vi "Periodic Tasks.vi"(8 "error in":errorcluster) -> ()   [LabVIEW 2020]
doc: "This VI runs in parallel to other tasks. It can contain as many user-defined periodic loops as you need. These can carry out PID or other sorts of timed response."
uses:
  <vilib>/Rock Robotics/WPI/ThirdParty/Phoenix-LabVIEW/Motor Controller/Controls/CTRE_Phoenix_MotorControl_ControlMode.ctl
  <vilib>/Rock Robotics/WPI/Solenoid/WPI_SolenoidValue.ctl
  <vilib>/Rock Robotics/WPI/DriverStation/WPI_DriverStationAllianceInfo.ctl
  <vilib>/Rock Robotics/WPI/Utilities/WPI_GetSetVariantRefNum.vi
  Robot Global Data.vi
  <vilib>/Rock Robotics/WPI/Solenoid/WPI_SolenoidSetEnum.vi
  <vilib>/Rock Robotics/WPI/ThirdParty/Phoenix-LabVIEW/Motor Controller/Get/CTRE_Phoenix_MotorController_IntegratedSensorData_TalonFX.vi
  <vilib>/Rock Robotics/WPI/ThirdParty/Phoenix-LabVIEW/Motor Controller/Get/CTRE_Phoenix_MotorController_GetQuadratureData.vi
  <vilib>/Rock Robotics/WPI/ThirdParty/Phoenix-LabVIEW/Motor Controller/Sensor/CTRE_Phoenix_MotorControl_SetIntegratedSensorPosition_TalonFX.vi
  <vilib>/Rock Robotics/Network Tables/NT Read Numeric Array.vi
  <vilib>/Rock Robotics/Network Tables/NT Read String Array.vi
  <vilib>/Rock Robotics/Network Tables/NT Read Boolean Array.vi
  <vilib>/Rock Robotics/Network Tables/NT Write String Array.vi
  <vilib>/Rock Robotics/Network Tables/NT Write Boolean Array.vi
  <vilib>/Rock Robotics/Network Tables/NT Write Numeric Array.vi
  <vilib>/Rock Robotics/Network Tables/NT Read Number.vi
  <vilib>/Rock Robotics/Network Tables/NT Write Number.vi
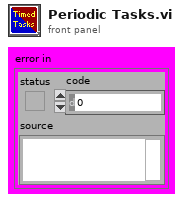
[diagram p1: front panel]
types:
  T1 = enum16{"Do Nothing", "Cargo", "Low", "High", "Long Shot", "U", "Hook", "Tee", "Eject"}
  T2 = enum16{"Do Nothing", "Cargo", "Low", "High", "Long Shot", "U", "Hook", "Tee"}
  T3 = typedef "WPI_GyroDevRef.ctl" = cluster{"DevStatus":errorcluster, "Analog Channel":T4, "Gain (VoltsPerDegree/Second)":dbl, "Gyro Type":enum16{"Analog", "XRS450"}, "Handle":i32, "SPI Bus":T5, "Device Found":bool, "Sample Rate":dbl, "Calibrate On Open":bool, "Offset":dbl}
  T4 = typedef "FPGA_AIChannel.ctl" = enum8{"AI 0", "AI 1", "AI 2", "AI 3", "AI MXP 0", "AI MXP 1", "AI MXP 2", "AI MXP 3", "Invalid"}
  T5 = typedef "spi_bus.ctl" = enum16{"SPI On-Board, CS0", "SPI On-Board, CS1", "SPI On-Board, CS2", "SPI On-Board, CS3", "SPI MXP", "Invalid"}
  T6 = typedef "WPI_PotentiometerDevRef.ctl" = cluster{"DevStatus":errorcluster, "Analog Channel":T4, "Invert Output":bool}
  T7 = typedef "WPI_DigitalInputDevRef.ctl" = cluster{"DevStatus":errorcluster, "DIO Channel":T8}
  T8 = typedef "FPGA_DIOChannel.ctl" = enum8{"DIO 0", "DIO 1", "DIO 2", "DIO 3", "DIO 4", "DIO 5", "DIO 6", "DIO 7", "DIO 8", "DIO 9", "DIO MXP 0", "DIO MXP 1", "DIO MXP 2", "DIO MXP 3", "DIO MXP 4", "DIO MXP 5", "DIO MXP 6", "DIO MXP 7", "DIO MXP 8", "DIO MXP 9", "DIO MXP 10", "DIO MXP 11", "DIO MXP 12", "DIO MXP 13", "DIO MXP 14", "DIO MXP 15", "SPI Port CS1", "SPI Port CS2", "SPI Port CS3", "SPI Port MISO", "SPI Port MOSI", "Invalid"}
  T9 = typedef "WPI_SolenoidDevRef.ctl" = cluster{"DevStatus":errorcluster, "Pneumatics Control Module":u8, "Forward Solenoid Channel":T10, "Reverse Solenoid Channel":T10}
  T10 = typedef "WPI_SolenoidChannel.ctl" = enum8{"Solenoid 0", "Solenoid 1", "Solenoid 2", "Solenoid 3", "Solenoid 4", "Solenoid 5", "Solenoid 6", "Solenoid 7", "Solenoid 8", "Solenoid 9", "Solenoid 10", "Solenoid 11", "Solenoid 12", "Solenoid 13", "Solenoid 14", "Solenoid 15", "Invalid"}
  T11 = typedef "WPI_SolenoidValue.ctl" = enum16{"Off", "On", "Forward", "Reverse"}
  T12 = typedef "WPI_AnalogChannelDevRef.ctl" = cluster{"DevStatus":errorcluster, "Analog Channel":T4}
  T13 = typedef "WPI_JoystickDevRef.ctl" = cluster{"Device":T14}
  T14 = typedef "WPI_JoystickDeviceEnum.ctl" = enum16{"USB 0", "USB 1", "USB 2", "USB 3", "USB 4", "USB 5"}
  T15 = typedef "WPI_MotorControlDeviceRef.ctl" = cluster{"DeviceStatus":errorcluster, "Type":T16, "PWM":cluster{"PWM Channel":T17, "DeadBand":T18}, "CAN":cluster{"Device Number":u8, "SetOutput VI Ref":variant, "GetOutput VI Ref":variant, "Enable VI Ref":variant, "Disable VI Ref":variant, "Data":variant}, "Invert":bool, "DIO PWM":cluster{"PWM \"Enable\" Channel":T17, "DIOChannel":T8, "PWM Rate":dbl}}
  T16 = typedef "WPI_MotorControlType.ctl" = enum16{"PWM", "CAN", "DIO PWM"}
  T17 = typedef "FPGA_DIOPWMChannel.ctl" = enum8{"PWM 0", "PWM 1", "PWM 2", "PWM 3", "PWM 4", "PWM 5", "PWM 6", "PWM 7", "PWM 8", "PWM 9", "PWM MXP 0", "PWM MXP 1", "PWM MXP 2", "PWM MXP 3", "PWM MXP 4", "PWM MXP 5", "PWM MXP 6", "PWM MXP 7", "PWM MXP 8", "PWM MXP 9", "Invalid"}
  T18 = typedef "WPI_PWMDeadband.ctl" = cluster{"Name":string, "maxPositivePwm":i32, "minPositivePwm":i32, "centerPwm":i32, "maxNegativePwm":i32, "minNegativePwm":i32, "angularRange":u16}
  T19 = typedef "CTRE_Phoenix_MotorControl_ControlMode.ctl" = u16
  T20 = typedef "WPI_RobotDriveDevRef.ctl" = cluster{"DevStatus":errorcluster, "Motors[]":T15[], "Square Inputs":bool, "Max Output":dbl}
  T21 = cluster{"JoystickDevRef":T13, "RobotDriveDevRef":T20}
  T22 = typedef "WPI_DigitalOutputDevRef.ctl" = cluster{"DIO Channel":T8, "DevStatus":errorcluster}
  T23 = typedef "WPI_DriverStationAllianceInfo.ctl" = enum16{"Red", "Blue", "Invalid"}
  T24 = typedef "WPI_RelayDevRef.ctl" = cluster{"DevStatus":errorcluster, "Relay Channel":T25, "Relay Direction":T26}
  T25 = typedef "FPGA_DIORelayChannel.ctl" = enum8{"Relay 0", "Relay 1", "Relay 2", "Relay 3", "Invalid"}
  T26 = typedef "WPI_RelayDirection.ctl" = enum16{"Both directions", "Forward only", "Reverse only"}
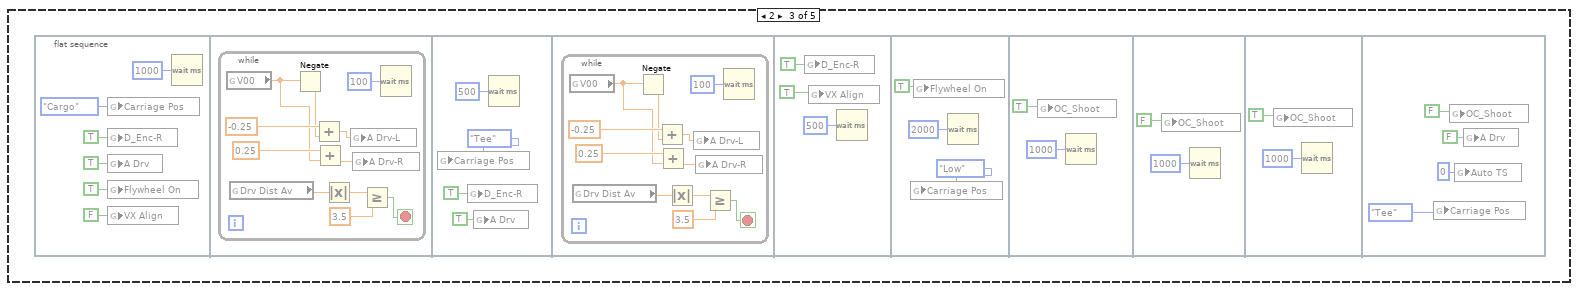
[diagram p13: hidden frame]
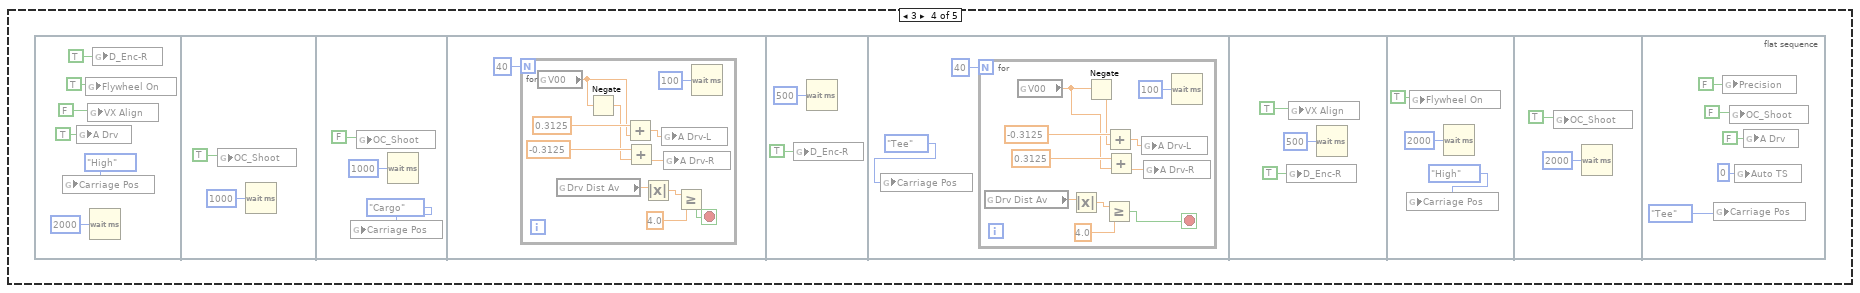
[diagram p14: hidden frame]
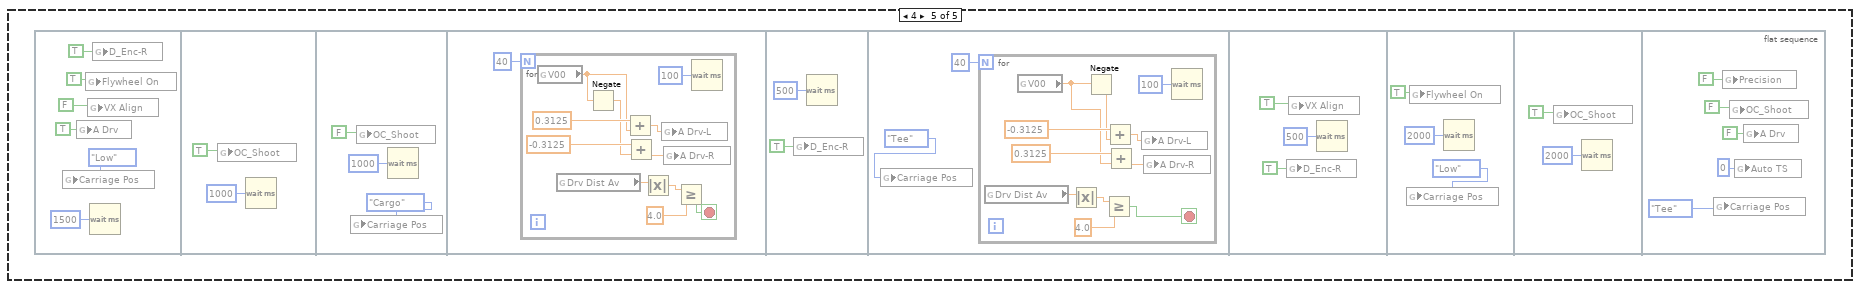
[diagram p15: hidden frame]
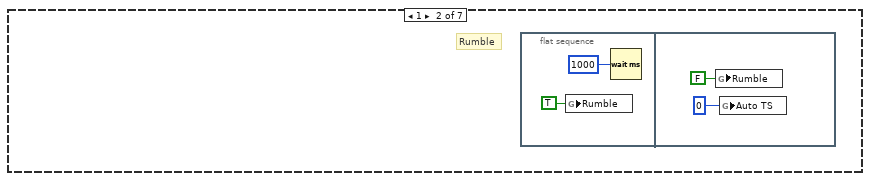
[diagram p18: hidden frame]
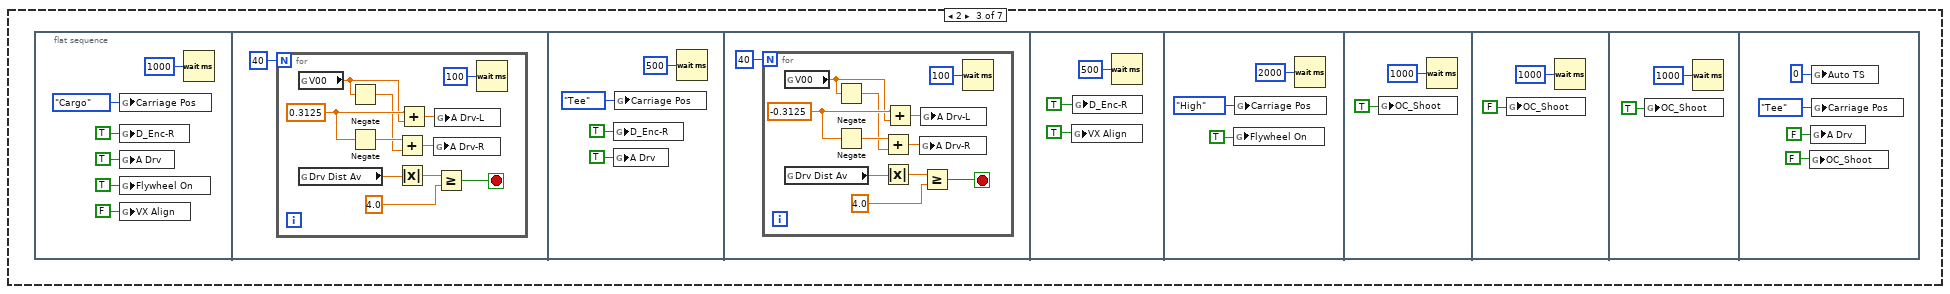
[diagram p19: hidden frame]
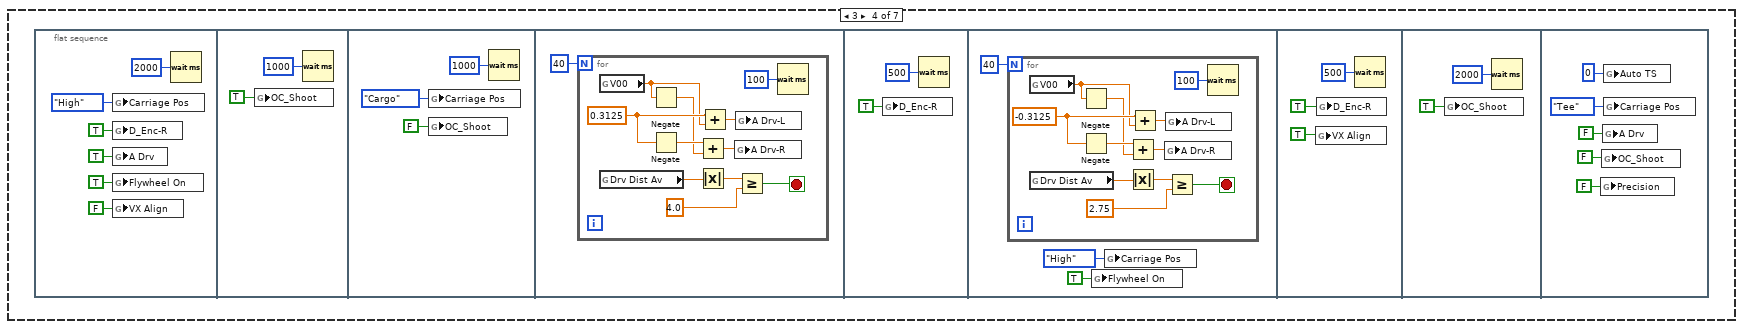
[diagram p20: hidden frame]
diagram:
  (unwired) "This VI is a good place to take care of periodic tasks such as control loops.\n\nAdd code to the existing loops, or duplicate a loop to define a new rate. You can allocate I/O references here, or in Begin.vi.\n\nPeriodic loops will often operate with setpoints from other loops. Use a global variable such as Robot Global Data for sharing data between loops."
  # "Autonomous\nTiming Sequence\n[Precondition: Tee Position]\n2 - Prep to pickup Cargo \nMove out of Tarmac to get one Cargo \nMove back into Tarmac to initial position \nMake two High Shots\n\n[Precondition: U Position]\n3 - Move to High position;\nMake one High Shot \nPrep to pickup Cargo \nMove out of  Tarmac to get one Cargo \nMove back into Tarmac to initial position  \nMake one High Shot\n\n[Precondition: U or Low Position]\n4 - Move to Low Position \nMake one Low Shot \nPrep to pickup Cargo \nMove out of Tarmac to get one Cargo \nMove back into Tarmac to initial position\nMake one Low Shot"
  # "Old Autonomous Sequences;\nStill works just is messy"
  # "s"
  n1 = disable-structure shown="Disabled" {
    frame Disabled {
      n2 = while {
        stop <- FALSE stop-if-true
        # "Autonomous\nTiming Sequence\n0 - Do Nothing\n1 - Rumble"
        n3 = global read "Robot Global Data.vi" "Auto TS"() -> (w39:i8)
        n4 = case shown="1" w39 {
          frame 0, Default {
            # "Do Nothing"
          }
          frame 1 {
            # "Rumble"
            n5 = flat-sequence {
              frame #0 {
                n6 = global write "Robot Global Data.vi" "Rumble"(TRUE ("Rumble")) -> ()
                n7 = Wait (ms)(milliseconds to wait=u32 1000) -> ()  [unwired: 1 out]
              }
              frame #1 {
                n8 = global write "Robot Global Data.vi" "Rumble"(FALSE ("Rumble")) -> ()
                n9 = global write "Robot Global Data.vi" "Auto TS"(i8 0 ("Autono R")) -> ()
              }
            }
          }
          frame 2 {
            n10 = flat-sequence {
              frame #0 {
                n11 = global write "Robot Global Data.vi" "Carriage Pos"(T1."Cargo" ("Carriage Pos")) -> ()
                n12 = global write "Robot Global Data.vi" "D_Enc-R"(TRUE ("D_Enc-R")) -> ()
                n13 = global write "Robot Global Data.vi" "A Drv"(TRUE ("A Drv")) -> ()
                n14 = global write "Robot Global Data.vi" "Flywheel On"(TRUE ("A Drv")) -> ()
                n15 = global write "Robot Global Data.vi" "VX Align"(FALSE ("VX Align")) -> ()
                n16 = Wait (ms)(milliseconds to wait=u32 1000) -> ()  [unwired: 1 out]
              }
              frame #1 {
                n17 = while {
                  stop <- w62 stop-if-true
                  n18 = global read "Robot Global Data.vi" "V00"() -> (w54:dbl)
                  n19 = global read "Robot Global Data.vi" "Drv Dist Av"() -> (w61:dbl)
                  n20 = Negate(x=w54) -> (-x=w53:dbl)
                  n21 = Add(x=-0.25 ("A Drv-L"), y=w53) -> (x+y=w58:dbl)
                  n22 = Add(x=0.25 ("A Drv-R"), y=w54) -> (x+y=w57:dbl)
                  n23 = Absolute Value(x=w61) -> (abs(x)=w52:dbl)
                  n24 = global write "Robot Global Data.vi" "A Drv-L"(w58) -> ()
                  n25 = global write "Robot Global Data.vi" "A Drv-R"(w57) -> ()
                  n26 = Greater Or Equal?(x=w52, y=3.5) -> (x >= y?=w62:bool)
                  n27 = Wait (ms)(milliseconds to wait=u32 100) -> ()  [unwired: 1 out]
                }
              }
              frame #2 {
                n28 = global write "Robot Global Data.vi" "Carriage Pos"(T2."Tee" ("Carriage Pos")) -> ()
                n29 = global write "Robot Global Data.vi" "D_Enc-R"(TRUE ("D_Enc-R")) -> ()
                n30 = global write "Robot Global Data.vi" "A Drv"(TRUE ("A Drv")) -> ()
                n31 = Wait (ms)(milliseconds to wait=u32 500) -> ()  [unwired: 1 out]
              }
              frame #3 {
                n32 = while {
                  stop <- w77 stop-if-true
                  n33 = global read "Robot Global Data.vi" "V00"() -> (w69:dbl)
                  n34 = global read "Robot Global Data.vi" "Drv Dist Av"() -> (w76:dbl)
                  n35 = Negate(x=w69) -> (-x=w68:dbl)
                  n36 = Add(x=-0.25 ("A Drv-L"), y=w68) -> (x+y=w73:dbl)
                  n37 = Add(x=0.25 ("A Drv-R"), y=w69) -> (x+y=w72:dbl)
                  n38 = Absolute Value(x=w76) -> (abs(x)=w67:dbl)
                  n39 = global write "Robot Global Data.vi" "A Drv-L"(w73) -> ()
                  n40 = global write "Robot Global Data.vi" "A Drv-R"(w72) -> ()
                  n41 = Greater Or Equal?(x=w67, y=3.5) -> (x >= y?=w77:bool)
                  n42 = Wait (ms)(milliseconds to wait=u32 100) -> ()  [unwired: 1 out]
                }
              }
              frame #4 {
                n43 = global write "Robot Global Data.vi" "D_Enc-R"(TRUE ("D_Enc-R")) -> ()
                n44 = global write "Robot Global Data.vi" "VX Align"(TRUE ("A Drv")) -> ()
                n45 = Wait (ms)(milliseconds to wait=u32 500) -> ()  [unwired: 1 out]
              }
              frame #5 {
                n46 = global write "Robot Global Data.vi" "Carriage Pos"(T2."Low" ("Carriage Pos")) -> ()
                n47 = global write "Robot Global Data.vi" "Flywheel On"(TRUE ("A Drv")) -> ()
                n48 = Wait (ms)(milliseconds to wait=u32 2000) -> ()  [unwired: 1 out]
              }
              frame #6 {
                n49 = global write "Robot Global Data.vi" "OC_Shoot"(TRUE ("A Drv")) -> ()
                n50 = Wait (ms)(milliseconds to wait=u32 1000) -> ()  [unwired: 1 out]
              }
              frame #7 {
                n51 = global write "Robot Global Data.vi" "OC_Shoot"(FALSE ("A Drv")) -> ()
                n52 = Wait (ms)(milliseconds to wait=u32 1000) -> ()  [unwired: 1 out]
              }
              frame #8 {
                n53 = global write "Robot Global Data.vi" "OC_Shoot"(TRUE ("A Drv")) -> ()
                n54 = Wait (ms)(milliseconds to wait=u32 1000) -> ()  [unwired: 1 out]
              }
              frame #9 {
                n55 = global write "Robot Global Data.vi" "Carriage Pos"(T2."Tee" ("Carriage Pos")) -> ()
                n56 = global write "Robot Global Data.vi" "OC_Shoot"(FALSE ("A Drv")) -> ()
                n57 = global write "Robot Global Data.vi" "Auto TS"(i8 0 ("Auto TS")) -> ()
                n58 = global write "Robot Global Data.vi" "A Drv"(FALSE ("A Drv")) -> ()
              }
            }
          }
          frame 3 {
            n59 = flat-sequence {
              frame #0 {
                n60 = global write "Robot Global Data.vi" "Carriage Pos"(T2."High" ("Carriage Pos")) -> ()
                n61 = global write "Robot Global Data.vi" "A Drv"(TRUE ("A Drv")) -> ()
                n62 = global write "Robot Global Data.vi" "Flywheel On"(TRUE ("A Drv")) -> ()
                n63 = global write "Robot Global Data.vi" "VX Align"(FALSE ("A Drv")) -> ()
                n64 = Wait (ms)(milliseconds to wait=u32 2000) -> ()  [unwired: 1 out]
                n65 = global write "Robot Global Data.vi" "D_Enc-R"(TRUE ("D_Enc-R")) -> ()
              }
              frame #1 {
                n66 = global write "Robot Global Data.vi" "OC_Shoot"(TRUE ("A Drv")) -> ()
                n67 = Wait (ms)(milliseconds to wait=u32 1000) -> ()  [unwired: 1 out]
              }
              frame #2 {
                n68 = global write "Robot Global Data.vi" "Carriage Pos"(T2."Cargo" ("Carriage Pos")) -> ()
                n69 = global write "Robot Global Data.vi" "OC_Shoot"(FALSE ("A Drv")) -> ()
                n70 = Wait (ms)(milliseconds to wait=u32 1000) -> ()  [unwired: 1 out]
              }
              frame #3 {
                n71 = for {
                  N: 40 -> [_]
                  stop <- w106 stop-if-true
                  n72 = global read "Robot Global Data.vi" "V00"() -> (w109:dbl)
                  n73 = global read "Robot Global Data.vi" "Drv Dist Av"() -> (w108:dbl)
                  n74 = Negate(x=w109) -> (-x=w110:dbl)
                  n75 = Add(x=0.3125 ("A Drv-L"), y=w109) -> (x+y=w114:dbl)
                  n76 = Add(x=-0.3125 ("A Drv-R"), y=w110) -> (x+y=w113:dbl)
                  n77 = Absolute Value(x=w108) -> (abs(x)=w107:dbl)
                  n78 = global write "Robot Global Data.vi" "A Drv-L"(w114) -> ()
                  n79 = global write "Robot Global Data.vi" "A Drv-R"(w113) -> ()
                  n80 = Greater Or Equal?(x=w107, y=4.0) -> (x >= y?=w106:bool)
                  n81 = Wait (ms)(milliseconds to wait=u32 100) -> ()  [unwired: 1 out]
                }
              }
              frame #4 {
                n82 = global write "Robot Global Data.vi" "D_Enc-R"(TRUE ("D_Enc-R")) -> ()
                n83 = Wait (ms)(milliseconds to wait=u32 500) -> ()  [unwired: 1 out]
              }
              frame #5 {
                n84 = global write "Robot Global Data.vi" "Carriage Pos"(T2."Tee" ("Carriage Pos")) -> ()
                n85 = for {
                  N: 40 -> [_]
                  stop <- w121 stop-if-true
                  n86 = global read "Robot Global Data.vi" "Drv Dist Av"() -> (w123:dbl)
                  n87 = global read "Robot Global Data.vi" "V00"() -> (w126:dbl)
                  n88 = Absolute Value(x=w123) -> (abs(x)=w122:dbl)
                  n89 = Negate(x=w126) -> (-x=w125:dbl)
                  n90 = Greater Or Equal?(x=w122, y=4.0) -> (x >= y?=w121:bool)
                  n91 = Add(x=-0.3125 ("A Drv-L"), y=w125) -> (x+y=w130:dbl)
                  n92 = Add(x=0.3125 ("A Drv-R"), y=w126) -> (x+y=w129:dbl)
                  n93 = global write "Robot Global Data.vi" "A Drv-L"(w130) -> ()
                  n94 = global write "Robot Global Data.vi" "A Drv-R"(w129) -> ()
                  n95 = Wait (ms)(milliseconds to wait=u32 100) -> ()  [unwired: 1 out]
                }
              }
              frame #6 {
                n96 = global write "Robot Global Data.vi" "D_Enc-R"(TRUE ("D_Enc-R")) -> ()
                n97 = global write "Robot Global Data.vi" "VX Align"(TRUE ("A Drv")) -> ()
                n98 = Wait (ms)(milliseconds to wait=u32 500) -> ()  [unwired: 1 out]
              }
              frame #7 {
                n99 = global write "Robot Global Data.vi" "Carriage Pos"(T2."High" ("Carriage Pos")) -> ()
                n100 = global write "Robot Global Data.vi" "Flywheel On"(TRUE ("A Drv")) -> ()
                n101 = Wait (ms)(milliseconds to wait=u32 2000) -> ()  [unwired: 1 out]
              }
              frame #8 {
                n102 = global write "Robot Global Data.vi" "OC_Shoot"(TRUE ("A Drv")) -> ()
                n103 = Wait (ms)(milliseconds to wait=u32 2000) -> ()  [unwired: 1 out]
              }
              frame #9 {
                n104 = global write "Robot Global Data.vi" "Carriage Pos"(T2."Tee" ("Carriage Pos")) -> ()
                n105 = global write "Robot Global Data.vi" "Precision"(FALSE ("Precision")) -> ()
                n106 = global write "Robot Global Data.vi" "OC_Shoot"(FALSE ("A Drv")) -> ()
                n107 = global write "Robot Global Data.vi" "Auto TS"(i8 0 ("Auto TS")) -> ()
                n108 = global write "Robot Global Data.vi" "A Drv"(FALSE ("A Drv")) -> ()
              }
            }
          }
          frame 4 {
            n109 = flat-sequence {
              frame #0 {
                n110 = global write "Robot Global Data.vi" "Carriage Pos"(T2."Low" ("Carriage Pos")) -> ()
                n111 = global write "Robot Global Data.vi" "A Drv"(TRUE ("A Drv")) -> ()
                n112 = global write "Robot Global Data.vi" "Flywheel On"(TRUE ("A Drv")) -> ()
                n113 = global write "Robot Global Data.vi" "VX Align"(FALSE ("A Drv")) -> ()
                n114 = Wait (ms)(milliseconds to wait=u32 1500) -> ()  [unwired: 1 out]
                n115 = global write "Robot Global Data.vi" "D_Enc-R"(TRUE ("D_Enc-R")) -> ()
              }
              frame #1 {
                n116 = global write "Robot Global Data.vi" "OC_Shoot"(TRUE ("A Drv")) -> ()
                n117 = Wait (ms)(milliseconds to wait=u32 1000) -> ()  [unwired: 1 out]
              }
              frame #2 {
                n118 = global write "Robot Global Data.vi" "Carriage Pos"(T2."Cargo" ("Carriage Pos")) -> ()
                n119 = global write "Robot Global Data.vi" "OC_Shoot"(FALSE ("A Drv")) -> ()
                n120 = Wait (ms)(milliseconds to wait=u32 1000) -> ()  [unwired: 1 out]
              }
              frame #3 {
                n121 = for {
                  N: 40 -> [_]
                  stop <- w157 stop-if-true
                  n122 = global read "Robot Global Data.vi" "V00"() -> (w160:dbl)
                  n123 = global read "Robot Global Data.vi" "Drv Dist Av"() -> (w159:dbl)
                  n124 = Negate(x=w160) -> (-x=w161:dbl)
                  n125 = Add(x=0.3125 ("A Drv-L"), y=w160) -> (x+y=w165:dbl)
                  n126 = Add(x=-0.3125 ("A Drv-R"), y=w161) -> (x+y=w164:dbl)
                  n127 = Absolute Value(x=w159) -> (abs(x)=w158:dbl)
                  n128 = global write "Robot Global Data.vi" "A Drv-L"(w165) -> ()
                  n129 = global write "Robot Global Data.vi" "A Drv-R"(w164) -> ()
                  n130 = Greater Or Equal?(x=w158, y=4.0) -> (x >= y?=w157:bool)
                  n131 = Wait (ms)(milliseconds to wait=u32 100) -> ()  [unwired: 1 out]
                }
              }
              frame #4 {
                n132 = global write "Robot Global Data.vi" "D_Enc-R"(TRUE ("D_Enc-R")) -> ()
                n133 = Wait (ms)(milliseconds to wait=u32 500) -> ()  [unwired: 1 out]
              }
              frame #5 {
                n134 = global write "Robot Global Data.vi" "Carriage Pos"(T2."Tee" ("Carriage Pos")) -> ()
                n135 = for {
                  N: 40 -> [_]
                  stop <- w172 stop-if-true
                  n136 = global read "Robot Global Data.vi" "Drv Dist Av"() -> (w174:dbl)
                  n137 = global read "Robot Global Data.vi" "V00"() -> (w177:dbl)
                  n138 = Absolute Value(x=w174) -> (abs(x)=w173:dbl)
                  n139 = Negate(x=w177) -> (-x=w176:dbl)
                  n140 = Greater Or Equal?(x=w173, y=4.0) -> (x >= y?=w172:bool)
                  n141 = Add(x=-0.3125 ("A Drv-L"), y=w176) -> (x+y=w181:dbl)
                  n142 = Add(x=0.3125 ("A Drv-R"), y=w177) -> (x+y=w180:dbl)
                  n143 = global write "Robot Global Data.vi" "A Drv-L"(w181) -> ()
                  n144 = global write "Robot Global Data.vi" "A Drv-R"(w180) -> ()
                  n145 = Wait (ms)(milliseconds to wait=u32 100) -> ()  [unwired: 1 out]
                }
              }
              frame #6 {
                n146 = global write "Robot Global Data.vi" "D_Enc-R"(TRUE ("D_Enc-R")) -> ()
                n147 = global write "Robot Global Data.vi" "VX Align"(TRUE ("A Drv")) -> ()
                n148 = Wait (ms)(milliseconds to wait=u32 500) -> ()  [unwired: 1 out]
              }
              frame #7 {
                n149 = global write "Robot Global Data.vi" "Carriage Pos"(T2."Low" ("Carriage Pos")) -> ()
                n150 = global write "Robot Global Data.vi" "Flywheel On"(TRUE ("A Drv")) -> ()
                n151 = Wait (ms)(milliseconds to wait=u32 2000) -> ()  [unwired: 1 out]
              }
              frame #8 {
                n152 = global write "Robot Global Data.vi" "OC_Shoot"(TRUE ("A Drv")) -> ()
                n153 = Wait (ms)(milliseconds to wait=u32 2000) -> ()  [unwired: 1 out]
              }
              frame #9 {
                n154 = global write "Robot Global Data.vi" "Carriage Pos"(T2."Tee" ("Carriage Pos")) -> ()
                n155 = global write "Robot Global Data.vi" "Precision"(FALSE ("Precision")) -> ()
                n156 = global write "Robot Global Data.vi" "OC_Shoot"(FALSE ("A Drv")) -> ()
                n157 = global write "Robot Global Data.vi" "Auto TS"(i8 0 ("Auto TS")) -> ()
                n158 = global write "Robot Global Data.vi" "A Drv"(FALSE ("A Drv")) -> ()
              }
            }
          }
        }
        n159 = Wait (ms)(milliseconds to wait=u32 100) -> ()  [unwired: 1 out]
      }
    }
    frame Enabled {
    }
  }
  n160 = disable-structure shown="Disabled" {
    frame Disabled {
      n161 = while {
        stop <- FALSE stop-if-true
        n162 = global read "Robot Global Data.vi" "Backup"() -> (w196:bool)
        n163 = case shown="True" w196 {
          frame False {
          }
          frame True {
            n164 = flat-sequence {
              frame #0 {
                n165 = global write "Robot Global Data.vi" "A Drv"(TRUE ("A Drv")) -> ()
                n166 = Wait (ms)(milliseconds to wait=u32 250) -> ()  [unwired: 1 out]
              }
              frame #1 {
                n167 = while {
                  stop <- w211 stop-if-true
                  n168 = global read "Robot Global Data.vi" "Drv Dist Av"() -> (w202:dbl)
                  n169 = global read "Robot Global Data.vi" "V00"() -> (w203:dbl)
                  n170 = Add(x=0.3125 ("A Drv-L"), y=w203) -> (x+y=w208:dbl)
                  n171 = Negate(x=w203) -> (-x=w204:dbl)
                  n172 = Add(x=-0.3125 ("A Drv-R"), y=w204) -> (x+y=w207:dbl)
                  n173 = Absolute Value(x=w202) -> (abs(x)=w201:dbl)
                  n174 = global write "Robot Global Data.vi" "A Drv-L"(w208) -> ()
                  n175 = global write "Robot Global Data.vi" "A Drv-R"(w207) -> ()
                  n176 = Greater Or Equal?(x=w201, y=1.0) -> (x >= y?=w211:bool)
                  n177 = Wait (ms)(milliseconds to wait=u32 100) -> ()  [unwired: 1 out]
                }
              }
              frame #2 {
                n178 = global write "Robot Global Data.vi" "Backup"(FALSE ("Backup")) -> ()
                n179 = global write "Robot Global Data.vi" "OC_Align VX"(TRUE ("A Drv")) -> ()
                n180 = global write "Robot Global Data.vi" "D_Enc-R"(TRUE ("D_Enc-R")) -> ()
                n181 = global write "Robot Global Data.vi" "A Drv"(FALSE ("A Drv")) -> ()
                n182 = global write "Robot Global Data.vi" "A Drv-L"(0.0 ("A Drv-L")) -> ()
                n183 = global write "Robot Global Data.vi" "A Drv-R"(0.0 ("A Drv-R")) -> ()
              }
            }
          }
        }
        n184 = Wait (ms)(milliseconds to wait=u32 100) -> ()  [unwired: 1 out]
      }
    }
    frame Enabled {
    }
  }
  n185 = disable-structure shown="Disabled" {
    frame Disabled {
      n186 = call <vilib>:"WPI_GyroRefNum Registry Get.vi"("refnum name"="B_Gyro") -> ("GyroDevRef"=w218:T3)  [unwired: 9 in, 1 out]
      n187 = while {
        tunnel: w218 -> [w224]
        tunnel: [w223] -> _
        stop <- FALSE stop-if-true
        # "Gyro Compensation"
        # "Adds Gyro Comp"
        # "0 to 179 and -1 to -180"
        # "0-359"
        # "Gyro (AI 1)"
        n188 = global read "Robot Global Data.vi" "Gyro Reset"() -> (w225:bool)
        n189 = case shown="True" w225 {
          tunnel: w224 -> [w239 w242]
          tunnel: [w239 w241] -> w226
          frame False {
          }
          frame True {
            n190 = global write "Robot Global Data.vi" "Gyro Reset"(FALSE ("Encoder Reset")) -> ()
            n191 = global write "Robot Global Data.vi" "G Cal"(0.0 ("G Cal")) -> ()
            n192 = call <vilib>:"WPI_GyroReset.vi"("GyroDevRef"=w242) -> ("GyroDevRef"=w241:T3)  [unwired: 9 in, 1 out]
          }
        }
        n193 = call <vilib>:"WPI_GyroGetAngle.vi"("GyroDevRef"=w226) -> ("Angle"=w227:dbl, "GyroDevRef"=w223:T3)  [unwired: 6 in, 3 out]
        n194 = global read "Robot Global Data.vi" "G Cal"() -> (w229:dbl)
        n195 = Quotient & Remainder(x=w227, y=360.0) -> (x-y*floor(x/y)=w230:dbl)  [unwired: 1 out]
        n196 = Add(x=w230, y=w229) -> (x+y=w235:dbl)
        n197 = Less?(x=w235, y=180.0) -> (x < y?=w233:bool)
        n198 = Subtract(x=w235, y=360.0) -> (x-y=w234:dbl)
        n199 = Select(t=w235, s=w233, f=w234) -> (s? t:f=w236:dbl)
        n200 = global read "Robot Global Data.vi" "G Offset"() -> (w221:dbl)
        n201 = global read "Robot Global Data.vi" "G Cal"() -> (w220:dbl)
        n202 = global write "Robot Global Data.vi" "Gyro"(w236) -> ()
        n203 = Add(x=w221, y=w220) -> (x+y=w222:dbl)
        n204 = global write "Robot Global Data.vi" "G Cal"(w222) -> ()
        n205 = Wait (ms)(milliseconds to wait=u32 100) -> ()  [unwired: 1 out]
      }
    }
    frame Enabled {
    }
  }
  n206 = disable-structure shown="Disabled" {
    frame Disabled {
      n207 = call <vilib>:"WPI_PotentiometerRefNum Registry Get.vi"("refnum name"="B_Photo LS On") -> ("PotDevRef"=w246:T6)  [unwired: 9 in, 1 out]
      n208 = call <vilib>:"WPI_DigitalInputRefNum Registry Get.vi"("refnum name"="B_LS On") -> ("DigitalInputDevRef"=w244:T7)  [unwired: 9 in, 1 out]
      n209 = while {
        tunnel: w246 -> [w255]
        tunnel: [w254] -> _
        stop <- FALSE stop-if-true
        # "Changed 5 to 60"
        # "1000, 60"
        # "Photosensor (AI 0)"
        n210 = call <vilib>:"WPI_PotentiometerGetNormalized.vi"("PotDevRef"=w255) -> ("Normalized Value"=w258:dbl, "PotDevRef"=w254:T6)  [unwired: 8 in, 1 out]
        n211 = Multiply(x=w258, y=1000.0) -> (x*y=w256:dbl)
        n212 = Greater?(x=w256, y=60.0) -> (0:w259:bool)
        n213 = global write "Robot Global Data.vi" "Photo LS Num"(w256) -> ()
        n214 = global write "Robot Global Data.vi" "Photo LS On"(w259) -> ()
        n215 = Wait (ms)(milliseconds to wait=u32 100) -> ()  [unwired: 1 out]
      }
      n216 = while {
        tunnel: w244 -> [w251]
        tunnel: [w250] -> _
        stop <- FALSE stop-if-true
        # "Limit Switch (DIO 0)"
        n217 = call <vilib>:"WPI_DigitalInputGetValue.vi"("DigitalInputDevRef"=w251) -> ("Value"=w248:bool, "DigitalInputDevRef"=w250:T7)  [unwired: 8 in, 1 out]
        n218 = Not(x=w248) -> (.not. x?=w249:bool)
        n219 = global write "Robot Global Data.vi" "LS On"(w249) -> ()
        n220 = Wait (ms)(milliseconds to wait=u32 100) -> ()  [unwired: 1 out]
      }
    }
    frame Enabled {
    }
  }
  n221 = while {
    stop <- FALSE stop-if-true
    n222 = global read "Robot Global Data.vi" "OC_Shoot Off"() -> (w263:bool)
    n223 = case shown="True" w263 {
      frame False {
      }
      frame True {
        n224 = flat-sequence {
          frame #0 {
            n225 = Wait (ms)(milliseconds to wait=u32 3000) -> ()  [unwired: 1 out]
          }
          frame #1 {
            n226 = global write "Robot Global Data.vi" "OC_Shoot Off"(FALSE ("OC_Shoot Off")) -> ()
          }
        }
      }
    }
    n227 = Wait (ms)(milliseconds to wait=u32 100) -> ()  [unwired: 1 out]
  }
  n228 = call <vilib>:"WPI_SolenoidRefNum Registry Get.vi"("refnum name"="B_LA") -> ("SolenoidDevRef"=w22:T9)  [unwired: 9 in, 1 out]
  n229 = disable-structure shown="Disabled" {
    frame Disabled {
      # "if score >70  then Dash In View add to Dashboard"
      n230 = call-poly <vilib>:"NT Read Value.vi"("Name"="D_W Boolean Array") -> ("Boolean Array"=w270:bool[])  [unwired: 9 in, 1 out]
      n231 = Index Array(array=w270) -> (element=w268:bool)  [unwired: 1 in]
      n232 = global write "Robot Global Data.vi" "Dash In View"(w268) -> ()
      n233 = global read "Robot Global Data.vi" "Dash X"() -> ()  [unwired: 1 in]
      n234 = global read "Robot Global Data.vi" "Distance"() -> ()  [unwired: 1 in]
      n235 = global read "Robot Global Data.vi" "Score"() -> ()  [unwired: 1 in]
      n236 = global read "Robot Global Data.vi" "Dash Y"() -> ()  [unwired: 1 in]
    }
    frame Enabled {
    }
  }
  n237 = while {
    tunnel: w22 -> [w276]
    tunnel: [w275] -> _
    stop <- FALSE stop-if-true
    # "Trailing Bar Pistons"
    n238 = global read "Robot Global Data.vi" "TB_Out"() -> (w274:bool)
    n239 = Select(t=WPI_SolenoidValue."Reverse" ("Value"), s=w274, f=WPI_SolenoidValue."Forward" ("Value")) -> (s? t:f=w271:T11)
    n240 = call-poly <vilib>:"WPI_SolenoidSet.vi"("Value"=w271, "SolenoidDevRef"=w276) -> ("SolenoidDevRef"=w275:T9)  [unwired: 8 in, 1 out]
    n241 = Wait (ms)(milliseconds to wait=u32 100) -> ()  [unwired: 1 out]
  }
  n242 = disable-structure shown="Disabled" {
    frame Disabled {
      # "Just to find Global Vars;\n(ignore this)"
      n243 = global read "Robot Global Data.vi" "A Drv"() -> ()  [unwired: 1 out]
    }
    frame Enabled {
    }
  }
  n244 = call <vilib>:"WPI_AnalogChannelRefNum Registry Get.vi"("refnum name"="B_Tee Pot") -> ("AIDeviceRef"=w37:T12)  [unwired: 9 in, 1 out]
  n245 = call <vilib>:"WPI_DigitalInputRefNum Registry Get.vi"("refnum name"="B_Tee LS Hi") -> ("DigitalInputDevRef"=w33:T7)  [unwired: 9 in, 1 out]
  n246 = call <vilib>:"WPI_DigitalInputRefNum Registry Get.vi"("refnum name"="B_Tee LS Lo") -> ("DigitalInputDevRef"=w35:T7)  [unwired: 9 in, 1 out]
  n247 = call <vilib>:"WPI_SolenoidRefNum Registry Get.vi"("refnum name"="B_Tee") -> ("SolenoidDevRef"=w32:T9)  [unwired: 9 in, 1 out]
  n248 = call <vilib>:"WPI_JoystickRefNum Registry Get.vi"("refnum name"="B_Driver") -> ("JoystickDevRef"=w17:T13)  [unwired: 9 in, 1 out]
  n249 = call <vilib>:"WPI_JoystickRefNum Registry Get.vi"("refnum name"="B_Operator 1") -> ("JoystickDevRef"=w16:T13)  [unwired: 9 in, 1 out]
  n250 = call <vilib>:"CTRE_Phoenix_MotorControl_RefNumRegistryGet.vi"("refnum name"="B_Tee_L") -> ("PhoenixMotorControlDevRef"=w4:T15)  [unwired: 9 in, 1 out]
  n251 = call <vilib>:"CTRE_Phoenix_MotorControl_RefNumRegistryGet.vi"("refnum name"="B_Tee_R") -> ("PhoenixMotorControlDevRef"=w3:T15)  [unwired: 9 in, 1 out]
  n252 = disable-structure shown="Disabled" {
    frame Disabled {
      # "x1"
      n253 = call <vilib>:"CTRE_Phoenix_MotorControl_RefNumRegistryGet.vi"("refnum name"="B_Tee_L") -> ("PhoenixMotorControlDevRef"=w282:T15)  [unwired: 9 in, 1 out]
      n254 = call <vilib>:"CTRE_Phoenix_MotorControl_RefNumRegistryGet.vi"("refnum name"="B_Tee_R") -> ("PhoenixMotorControlDevRef"=w281:T15)  [unwired: 9 in, 1 out]
      n255 = while {
        tunnel: w282 -> [w326]
        tunnel: w281 -> [w325]
        tunnel: [w329] -> _
        tunnel: [w328] -> _
        stop <- FALSE stop-if-true
        w327 = T19 0 items=["PercentOutput"=0, "Position"=1, "Velocity"=2, "Current"=3, "Follower"=5, "MotionProfile"=6, "MotionMagic"=7, "MotionProfileArc"=10, "Disabled"=15] ("Control Mode")
        # "Rotational Thresholds"
        # "Tee/Carriage Driver"
        n256 = global read "Robot Global Data.vi" "OC_LA_Reset"() -> (w324:bool)
        n257 = global read "Robot Global Data.vi" "OC_Tee Pwr"() -> (w293:dbl)
        n258 = global read "Robot Global Data.vi" "DC Tee Pwr"() -> (w294:dbl)
        n259 = Absolute Value(x=w294) -> (abs(x)=w297:dbl)
        n260 = case shown="True" w324 {
          tunnel: w326 -> [w332 w338]
          tunnel: w325 -> [w331 w337]
          tunnel: [w332 w335] -> w323
          tunnel: [w331 w333] -> w322
          frame False {
          }
          frame True {
            n261 = flat-sequence {
              tunnel: w338 -> [w341]
              tunnel: w337 -> [w342]
              tunnel: [w340] -> w336
              tunnel: [w339] -> w334
              tunnel: [w346] -> w335
              tunnel: w336 -> [w346]
              tunnel: [w345] -> w333
              tunnel: w334 -> [w345]
              frame #0 {
                n262 = call <vilib>:"CTRE_Phoenix_MotorControl_SetSelectedSensorPosition.vi"("New Sensor Position"=0, "PhoenixMotorControlDevRef"=w342) -> ("PhoenixMotorControlDevRef"=w339:T15)  [unwired: 8 in, 1 out]
                n263 = call <vilib>:"CTRE_Phoenix_MotorControl_SetSelectedSensorPosition.vi"("New Sensor Position"=0, "PhoenixMotorControlDevRef"=w341) -> ("PhoenixMotorControlDevRef"=w340:T15)  [unwired: 8 in, 1 out]
              }
              frame #1 {
                n264 = global write "Robot Global Data.vi" "OC_LA_Reset"(FALSE ("OC_LA_Reset")) -> ()
              }
            }
          }
        }
        n265 = Greater?(x=w297, y=0.2) -> (0:w295:bool)
        n266 = Select(t=w294, s=w295, f=w293) -> (s? t:f=w289:dbl)
        n267 = Absolute Value(x=w289) -> (abs(x)=w292:dbl)
        n268 = Greater?(x=w292, y=0.2) -> (0:w290:bool)
        n269 = global read "Robot Global Data.vi" "Auto Tee Pwr"() -> (w287:dbl)
        n270 = global read "Robot Global Data.vi" "Climb On"() -> (w286:bool)
        n271 = Select(t=w289, s=w290, f=0.0) -> (s? t:f=w285:dbl)
        n272 = Select(t=w285, s=w286, f=w287) -> (s? t:f=w284:dbl)
        n273 = call-poly <vilib>:"CTRE_Phoenix_MotorController_Get_Enhanced.vi"("PhoenixMotorControlDevRef"=w323) -> ("PhoenixMotorControlDevRef"=w321:T15)  [unwired: 11 in, 3 out]
        n274 = call-poly <vilib>:"CTRE_Phoenix_MotorController_Get_Enhanced.vi"("PhoenixMotorControlDevRef"=w322) -> ("PhoenixMotorControlDevRef"=w320:T15)  [unwired: 11 in, 3 out]
        n275 = Negate(x=w284) -> (-x=w300:dbl)
        n276 = global read "Robot Global Data.vi" "Tee_Pot"() -> (w315:dbl)
        n277 = global read "Robot Global Data.vi" "Lo LS"() -> (w305:bool)
        n278 = Greater?(x=w315, y=330.0) -> (0:w304:bool)
        n279 = In Range and Coerce(upper limit=1.0, x=w300, lower limit=0.0) -> (coerced(x)=w317:dbl)  [unwired: 1 out]
        n280 = Or(x=w305, y=w304) -> (x .or. y?=w303:bool)
        n281 = Select(t=w317, s=w303, f=w300) -> (s? t:f=w309:dbl)
        n282 = global read "Robot Global Data.vi" "Tee_Pot"() -> (w310:dbl)
        n283 = global read "Robot Global Data.vi" "Hi LS"() -> (w306:bool)
        n284 = Less?(x=w310, y=160.0) -> (x < y?=w308:bool)
        n285 = In Range and Coerce(upper limit=0.0, x=w309, lower limit=-1.0) -> (coerced(x)=w312:dbl)  [unwired: 1 out]
        n286 = Or(x=w306, y=w308) -> (x .or. y?=w307:bool)
        n287 = Select(t=w312, s=w307, f=w309) -> (s? t:f=w302:dbl)
        n288 = Multiply(x=w302, y=0.55) -> (x*y=w298:dbl)
        n289 = Negate(x=w298) -> (-x=w299:dbl)
        n290 = call <vilib>:"CTRE_Phoenix_MotorControl_Set.vi"("Output"=w298, "Control Mode"=w327, "PhoenixMotorControlDevRef"=w321) -> ("PhoenixMotorControlDevRef"=w329:T15)  [unwired: 7 in, 1 out]
        n291 = call <vilib>:"CTRE_Phoenix_MotorControl_Set.vi"("Output"=w299, "Control Mode"=w327, "PhoenixMotorControlDevRef"=w320) -> ("PhoenixMotorControlDevRef"=w328:T15)  [unwired: 7 in, 1 out]
        n292 = Wait (ms)(milliseconds to wait=u32 100) -> ()  [unwired: 1 out]
      }
    }
    frame Enabled {
    }
  }
  n293 = while {
    tunnel: w32 -> [w353]
    tunnel: [w352] -> _
    stop <- FALSE stop-if-true
    n294 = global read "Robot Global Data.vi" "Tee-Out"() -> (w351:bool)
    n295 = Select(t=WPI_SolenoidValue."Reverse" ("Value"), s=w351, f=WPI_SolenoidValue."Forward" ("Value")) -> (s? t:f=w348:T11)
    n296 = call-poly <vilib>:"WPI_SolenoidSet.vi"("Value"=w348, "SolenoidDevRef"=w353) -> ("SolenoidDevRef"=w352:T9)  [unwired: 8 in, 1 out]
    n297 = Wait (ms)(milliseconds to wait=u32 100) -> ()  [unwired: 1 out]
  }
  n298 = while {
    tunnel: w37 -> [w359]
    tunnel: [w360] -> _
    stop <- FALSE stop-if-true
    n299 = call <vilib>:"WPI_AnalogChannelGetVoltage.vi"("AIDeviceRef"=w359) -> ("Voltage"=w356:dbl, "AIDeviceRef"=w360:T12)  [unwired: 8 in, 1 out]
    n300 = Multiply(x=w356, y=100.0) -> (x*y=w358:dbl)
    n301 = global write "Robot Global Data.vi" "Raw Tee Pot"(w356) -> ()
    n302 = global write "Robot Global Data.vi" "Tee_Pot"(w358) -> ()
    n303 = Wait (ms)(milliseconds to wait=u32 100) -> ()  [unwired: 1 out]
  }
  n304 = while {
    tunnel: w35 -> [w370]
    tunnel: [w369] -> _
    tunnel: w33 -> [w364]
    tunnel: [w363] -> _
    stop <- FALSE stop-if-true
    # "Limit Switch (DIO 0)"
    n305 = call <vilib>:"WPI_DigitalInputGetValue.vi"("DigitalInputDevRef"=w370) -> ("Value"=w367:bool, "DigitalInputDevRef"=w369:T7)  [unwired: 8 in, 1 out]
    n306 = call <vilib>:"WPI_DigitalInputGetValue.vi"("DigitalInputDevRef"=w364) -> ("Value"=w365:bool, "DigitalInputDevRef"=w363:T7)  [unwired: 8 in, 1 out]
    n307 = Not(x=w367) -> (.not. x?=w368:bool)
    n308 = Not(x=w365) -> (.not. x?=w366:bool)
    n309 = global write "Robot Global Data.vi" "Lo LS"(w368) -> ()
    n310 = global write "Robot Global Data.vi" "Hi LS"(w366) -> ()
    n311 = Wait (ms)(milliseconds to wait=u32 100) -> ()  [unwired: 1 out]
  }
  n312 = while {
    tunnel: w17 -> [w374]
    tunnel: w16 -> [w373]
    stop <- FALSE stop-if-true
    # "Rumble Driver Controller"
    n313 = global read "Robot Global Data.vi" "Rumble"() -> (w375:bool)
    n314 = case shown="True" w375 {
      tunnel: w374 -> [w380 w385]
      tunnel: w373 -> [w378 w382]
      frame False {
        w379 = sgl 0.0 ("Left Rumble")
        w381 = sgl 0.0 ("Left Rumble")
        n315 = call <vilib>:"WPI_JoystickSetOutputs.vi"("Right Rumble"=w381, "Left Rumble"=w381, "JoystickDevRef"=w380) -> ()  [unwired: 7 in, 2 out]
        n316 = call <vilib>:"WPI_JoystickSetOutputs.vi"("Right Rumble"=w379, "Left Rumble"=w379, "JoystickDevRef"=w378) -> ()  [unwired: 7 in, 2 out]
      }
      frame True {
        w383 = sgl 1.0 ("Left Rumble")
        w384 = sgl 1.0 ("Left Rumble")
        n317 = call <vilib>:"WPI_JoystickSetOutputs.vi"("Right Rumble"=w384, "Left Rumble"=w384, "JoystickDevRef"=w385) -> ()  [unwired: 7 in, 2 out]
        n318 = call <vilib>:"WPI_JoystickSetOutputs.vi"("Right Rumble"=w383, "Left Rumble"=w383, "JoystickDevRef"=w382) -> ()  [unwired: 7 in, 2 out]
      }
    }
    n319 = Wait (ms)(milliseconds to wait=u32 100) -> ()  [unwired: 1 out]
  }
  n320 = call <vilib>:"CTRE_Phoenix_MotorControl_RefNumRegistryGet.vi"("refnum name"="B_Belt") -> ("PhoenixMotorControlDevRef"=w27:T15)  [unwired: 9 in, 1 out]
  n321 = while {
    stop <- FALSE stop-if-true
    # "Autonomous\nTiming Sequence\n0 - Do Nothing\n1 - Rumble"
    n322 = global read "Robot Global Data.vi" "Auto TS"() -> (w388:i8)
    n323 = case shown="6" w388 {
      frame 0, Default {
      }
      frame 1 {
        # "Rumble"
        n324 = flat-sequence {
          frame #0 {
            n325 = global write "Robot Global Data.vi" "Rumble"(TRUE ("Rumble")) -> ()
            n326 = Wait (ms)(milliseconds to wait=u32 1000) -> ()  [unwired: 1 out]
          }
          frame #1 {
            n327 = global write "Robot Global Data.vi" "Rumble"(FALSE ("Rumble")) -> ()
            n328 = global write "Robot Global Data.vi" "Auto TS"(i8 0 ("Autono R")) -> ()
          }
        }
      }
      frame 2 {
        n329 = flat-sequence {
          frame #0 {
            n330 = global write "Robot Global Data.vi" "Carriage Pos"(T1."Cargo" ("Carriage Pos")) -> ()
            n331 = global write "Robot Global Data.vi" "D_Enc-R"(TRUE ("D_Enc-R")) -> ()
            n332 = global write "Robot Global Data.vi" "A Drv"(TRUE ("A Drv")) -> ()
            n333 = global write "Robot Global Data.vi" "Flywheel On"(TRUE ("A Drv")) -> ()
            n334 = global write "Robot Global Data.vi" "VX Align"(FALSE ("VX Align")) -> ()
            n335 = Wait (ms)(milliseconds to wait=u32 1000) -> ()  [unwired: 1 out]
          }
          frame #1 {
            n336 = for {
              N: 40 -> [_]
              stop <- w401 stop-if-true
              w404 = 0.3125 ("x")
              n337 = global read "Robot Global Data.vi" "V00"() -> (w403:dbl)
              n338 = global read "Robot Global Data.vi" "Drv Dist Av"() -> (w410:dbl)
              n339 = Negate(x=w403) -> (-x=w402:dbl)
              n340 = Negate(x=w404) -> (-x=w405:dbl)
              n341 = Add(x=w405, y=w402) -> (x+y=w407:dbl)
              n342 = Absolute Value(x=w410) -> (abs(x)=w409:dbl)
              n343 = Add(x=w404, y=w403) -> (x+y=w406:dbl)
              n344 = global write "Robot Global Data.vi" "A Drv-R"(w407) -> ()
              n345 = global write "Robot Global Data.vi" "A Drv-L"(w406) -> ()
              n346 = Greater Or Equal?(x=w409, y=4.0) -> (x >= y?=w401:bool)
              n347 = Wait (ms)(milliseconds to wait=u32 100) -> ()  [unwired: 1 out]
            }
          }
          frame #2 {
            n348 = global write "Robot Global Data.vi" "D_Enc-R"(TRUE ("D_Enc-R")) -> ()
            n349 = global write "Robot Global Data.vi" "A Drv"(TRUE ("A Drv")) -> ()
            n350 = global write "Robot Global Data.vi" "Carriage Pos"(T1."Tee" ("Carriage Pos")) -> ()
            n351 = Wait (ms)(milliseconds to wait=u32 500) -> ()  [unwired: 1 out]
          }
          frame #3 {
            n352 = for {
              N: 40 -> [_]
              stop <- w417 stop-if-true
              w420 = -0.3125 ("x")
              n353 = global read "Robot Global Data.vi" "V00"() -> (w419:dbl)
              n354 = global read "Robot Global Data.vi" "Drv Dist Av"() -> (w426:dbl)
              n355 = Negate(x=w419) -> (-x=w418:dbl)
              n356 = Negate(x=w420) -> (-x=w421:dbl)
              n357 = Add(x=w421, y=w418) -> (x+y=w423:dbl)
              n358 = Absolute Value(x=w426) -> (abs(x)=w425:dbl)
              n359 = Add(x=w420, y=w419) -> (x+y=w422:dbl)
              n360 = global write "Robot Global Data.vi" "A Drv-R"(w423) -> ()
              n361 = global write "Robot Global Data.vi" "A Drv-L"(w422) -> ()
              n362 = Greater Or Equal?(x=w425, y=4.0) -> (x >= y?=w417:bool)
              n363 = Wait (ms)(milliseconds to wait=u32 100) -> ()  [unwired: 1 out]
            }
          }
          frame #4 {
            n364 = global write "Robot Global Data.vi" "VX Align"(TRUE ("A Drv")) -> ()
            n365 = global write "Robot Global Data.vi" "D_Enc-R"(TRUE ("D_Enc-R")) -> ()
            n366 = Wait (ms)(milliseconds to wait=u32 500) -> ()  [unwired: 1 out]
          }
          frame #5 {
            n367 = global write "Robot Global Data.vi" "Flywheel On"(TRUE ("A Drv")) -> ()
            n368 = global write "Robot Global Data.vi" "Carriage Pos"(T1."High" ("Carriage Pos")) -> ()
            n369 = Wait (ms)(milliseconds to wait=u32 2000) -> ()  [unwired: 1 out]
          }
          frame #6 {
            n370 = global write "Robot Global Data.vi" "OC_Shoot"(TRUE ("A Drv")) -> ()
            n371 = Wait (ms)(milliseconds to wait=u32 1000) -> ()  [unwired: 1 out]
          }
          frame #7 {
            n372 = global write "Robot Global Data.vi" "OC_Shoot"(FALSE ("A Drv")) -> ()
            n373 = Wait (ms)(milliseconds to wait=u32 1000) -> ()  [unwired: 1 out]
          }
          frame #8 {
            n374 = global write "Robot Global Data.vi" "OC_Shoot"(TRUE ("A Drv")) -> ()
            n375 = Wait (ms)(milliseconds to wait=u32 1000) -> ()  [unwired: 1 out]
          }
          frame #9 {
            n376 = global write "Robot Global Data.vi" "OC_Shoot"(FALSE ("A Drv")) -> ()
            n377 = global write "Robot Global Data.vi" "A Drv"(FALSE ("A Drv")) -> ()
            n378 = global write "Robot Global Data.vi" "Auto TS"(i8 0 ("Auto TS")) -> ()
            n379 = global write "Robot Global Data.vi" "Carriage Pos"(T1."Tee" ("Carriage Pos")) -> ()
          }
        }
      }
      frame 3 {
        n380 = flat-sequence {
          frame #0 {
            n381 = global write "Robot Global Data.vi" "Carriage Pos"(T1."High" ("Carriage Pos")) -> ()
            n382 = global write "Robot Global Data.vi" "D_Enc-R"(TRUE ("D_Enc-R")) -> ()
            n383 = global write "Robot Global Data.vi" "A Drv"(TRUE ("A Drv")) -> ()
            n384 = global write "Robot Global Data.vi" "Flywheel On"(TRUE ("A Drv")) -> ()
            n385 = global write "Robot Global Data.vi" "VX Align"(FALSE ("VX Align")) -> ()
            n386 = Wait (ms)(milliseconds to wait=u32 2000) -> ()  [unwired: 1 out]
          }
          frame #1 {
            n387 = global write "Robot Global Data.vi" "OC_Shoot"(TRUE ("A Drv")) -> ()
            n388 = Wait (ms)(milliseconds to wait=u32 1000) -> ()  [unwired: 1 out]
          }
          frame #2 {
            n389 = global write "Robot Global Data.vi" "Carriage Pos"(T1."Cargo" ("Carriage Pos")) -> ()
            n390 = global write "Robot Global Data.vi" "OC_Shoot"(FALSE ("A Drv")) -> ()
            n391 = Wait (ms)(milliseconds to wait=u32 1000) -> ()  [unwired: 1 out]
          }
          frame #3 {
            n392 = for {
              N: 40 -> [_]
              stop <- w456 stop-if-true
              w459 = 0.3125 ("x")
              n393 = global read "Robot Global Data.vi" "V00"() -> (w458:dbl)
              n394 = global read "Robot Global Data.vi" "Drv Dist Av"() -> (w465:dbl)
              n395 = Negate(x=w458) -> (-x=w457:dbl)
              n396 = Negate(x=w459) -> (-x=w460:dbl)
              n397 = Add(x=w460, y=w457) -> (x+y=w462:dbl)
              n398 = Absolute Value(x=w465) -> (abs(x)=w464:dbl)
              n399 = Add(x=w459, y=w458) -> (x+y=w461:dbl)
              n400 = global write "Robot Global Data.vi" "A Drv-R"(w462) -> ()
              n401 = global write "Robot Global Data.vi" "A Drv-L"(w461) -> ()
              n402 = Greater Or Equal?(x=w464, y=4.0) -> (x >= y?=w456:bool)
              n403 = Wait (ms)(milliseconds to wait=u32 100) -> ()  [unwired: 1 out]
            }
          }
          frame #4 {
            n404 = global write "Robot Global Data.vi" "D_Enc-R"(TRUE ("D_Enc-R")) -> ()
            n405 = Wait (ms)(milliseconds to wait=u32 500) -> ()  [unwired: 1 out]
          }
          frame #5 {
            n406 = for {
              N: 40 -> [_]
              stop <- w472 stop-if-true
              w475 = -0.3125 ("x")
              n407 = global read "Robot Global Data.vi" "V00"() -> (w474:dbl)
              n408 = global read "Robot Global Data.vi" "Drv Dist Av"() -> (w481:dbl)
              n409 = Negate(x=w474) -> (-x=w473:dbl)
              n410 = Negate(x=w475) -> (-x=w476:dbl)
              n411 = Add(x=w476, y=w473) -> (x+y=w478:dbl)
              n412 = Absolute Value(x=w481) -> (abs(x)=w480:dbl)
              n413 = Add(x=w475, y=w474) -> (x+y=w477:dbl)
              n414 = global write "Robot Global Data.vi" "A Drv-R"(w478) -> ()
              n415 = global write "Robot Global Data.vi" "A Drv-L"(w477) -> ()
              n416 = Greater Or Equal?(x=w480, y=2.75) -> (x >= y?=w472:bool)
              n417 = Wait (ms)(milliseconds to wait=u32 100) -> ()  [unwired: 1 out]
            }
            n418 = global write "Robot Global Data.vi" "Flywheel On"(TRUE ("A Drv")) -> ()
            n419 = global write "Robot Global Data.vi" "Carriage Pos"(T1."High" ("Carriage Pos")) -> ()
          }
          frame #6 {
            n420 = global write "Robot Global Data.vi" "VX Align"(TRUE ("A Drv")) -> ()
            n421 = global write "Robot Global Data.vi" "D_Enc-R"(TRUE ("D_Enc-R")) -> ()
            n422 = Wait (ms)(milliseconds to wait=u32 500) -> ()  [unwired: 1 out]
          }
          frame #7 {
            n423 = global write "Robot Global Data.vi" "OC_Shoot"(TRUE ("A Drv")) -> ()
            n424 = Wait (ms)(milliseconds to wait=u32 2000) -> ()  [unwired: 1 out]
          }
          frame #8 {
            n425 = global write "Robot Global Data.vi" "Precision"(FALSE ("Precision")) -> ()
            n426 = global write "Robot Global Data.vi" "OC_Shoot"(FALSE ("A Drv")) -> ()
            n427 = global write "Robot Global Data.vi" "A Drv"(FALSE ("A Drv")) -> ()
            n428 = global write "Robot Global Data.vi" "Auto TS"(i8 0 ("Auto TS")) -> ()
            n429 = global write "Robot Global Data.vi" "Carriage Pos"(T1."Tee" ("Carriage Pos")) -> ()
          }
        }
      }
      frame 4 {
        n430 = flat-sequence {
          frame #0 {
            n431 = global write "Robot Global Data.vi" "Carriage Pos"(T1."Low" ("Carriage Pos")) -> ()
            n432 = global write "Robot Global Data.vi" "D_Enc-R"(TRUE ("D_Enc-R")) -> ()
            n433 = global write "Robot Global Data.vi" "A Drv"(TRUE ("A Drv")) -> ()
            n434 = global write "Robot Global Data.vi" "Flywheel On"(TRUE ("A Drv")) -> ()
            n435 = global write "Robot Global Data.vi" "VX Align"(FALSE ("VX Align")) -> ()
            n436 = Wait (ms)(milliseconds to wait=u32 1500) -> ()  [unwired: 1 out]
          }
          frame #1 {
            n437 = global write "Robot Global Data.vi" "OC_Shoot"(TRUE ("A Drv")) -> ()
            n438 = Wait (ms)(milliseconds to wait=u32 1000) -> ()  [unwired: 1 out]
          }
          frame #2 {
            n439 = global write "Robot Global Data.vi" "Carriage Pos"(T1."Cargo" ("Carriage Pos")) -> ()
            n440 = global write "Robot Global Data.vi" "OC_Shoot"(FALSE ("A Drv")) -> ()
            n441 = Wait (ms)(milliseconds to wait=u32 1000) -> ()  [unwired: 1 out]
          }
          frame #3 {
            n442 = for {
              N: 40 -> [_]
              stop <- w505 stop-if-true
              w508 = 0.3125 ("x")
              n443 = global read "Robot Global Data.vi" "V00"() -> (w507:dbl)
              n444 = global read "Robot Global Data.vi" "Drv Dist Av"() -> (w514:dbl)
              n445 = Negate(x=w507) -> (-x=w506:dbl)
              n446 = Negate(x=w508) -> (-x=w509:dbl)
              n447 = Add(x=w509, y=w506) -> (x+y=w511:dbl)
              n448 = Absolute Value(x=w514) -> (abs(x)=w513:dbl)
              n449 = Add(x=w508, y=w507) -> (x+y=w510:dbl)
              n450 = global write "Robot Global Data.vi" "A Drv-R"(w511) -> ()
              n451 = global write "Robot Global Data.vi" "A Drv-L"(w510) -> ()
              n452 = Greater Or Equal?(x=w513, y=4.0) -> (x >= y?=w505:bool)
              n453 = Wait (ms)(milliseconds to wait=u32 100) -> ()  [unwired: 1 out]
            }
          }
          frame #4 {
            n454 = global write "Robot Global Data.vi" "D_Enc-R"(TRUE ("D_Enc-R")) -> ()
            n455 = Wait (ms)(milliseconds to wait=u32 500) -> ()  [unwired: 1 out]
          }
          frame #5 {
            n456 = for {
              N: 40 -> [_]
              stop <- w520 stop-if-true
              w523 = -0.3125 ("x")
              n457 = global read "Robot Global Data.vi" "V00"() -> (w522:dbl)
              n458 = global read "Robot Global Data.vi" "Drv Dist Av"() -> (w529:dbl)
              n459 = Negate(x=w522) -> (-x=w521:dbl)
              n460 = Negate(x=w523) -> (-x=w524:dbl)
              n461 = Add(x=w524, y=w521) -> (x+y=w526:dbl)
              n462 = Absolute Value(x=w529) -> (abs(x)=w528:dbl)
              n463 = Add(x=w523, y=w522) -> (x+y=w525:dbl)
              n464 = global write "Robot Global Data.vi" "A Drv-R"(w526) -> ()
              n465 = global write "Robot Global Data.vi" "A Drv-L"(w525) -> ()
              n466 = Greater Or Equal?(x=w528, y=4.0) -> (x >= y?=w520:bool)
              n467 = Wait (ms)(milliseconds to wait=u32 100) -> ()  [unwired: 1 out]
            }
            n468 = global write "Robot Global Data.vi" "Carriage Pos"(T1."Tee" ("Carriage Pos")) -> ()
          }
          frame #6 {
            n469 = global write "Robot Global Data.vi" "VX Align"(TRUE ("A Drv")) -> ()
            n470 = global write "Robot Global Data.vi" "D_Enc-R"(TRUE ("D_Enc-R")) -> ()
            n471 = Wait (ms)(milliseconds to wait=u32 500) -> ()  [unwired: 1 out]
          }
          frame #7 {
            n472 = global write "Robot Global Data.vi" "Flywheel On"(TRUE ("A Drv")) -> ()
            n473 = global write "Robot Global Data.vi" "Carriage Pos"(T1."Low" ("Carriage Pos")) -> ()
            n474 = Wait (ms)(milliseconds to wait=u32 2000) -> ()  [unwired: 1 out]
          }
          frame #8 {
            n475 = global write "Robot Global Data.vi" "OC_Shoot"(TRUE ("A Drv")) -> ()
            n476 = Wait (ms)(milliseconds to wait=u32 2000) -> ()  [unwired: 1 out]
          }
          frame #9 {
            n477 = global write "Robot Global Data.vi" "Precision"(FALSE ("Precision")) -> ()
            n478 = global write "Robot Global Data.vi" "OC_Shoot"(FALSE ("A Drv")) -> ()
            n479 = global write "Robot Global Data.vi" "A Drv"(FALSE ("A Drv")) -> ()
            n480 = global write "Robot Global Data.vi" "Auto TS"(i8 0 ("Auto TS")) -> ()
            n481 = global write "Robot Global Data.vi" "Carriage Pos"(T1."Tee" ("Carriage Pos")) -> ()
          }
        }
      }
      frame 5 {
        n482 = flat-sequence {
          frame #0 {
            n483 = global write "Robot Global Data.vi" "Carriage Pos"(T1."High" ("Carriage Pos")) -> ()
            n484 = global write "Robot Global Data.vi" "D_Enc-R"(TRUE ("D_Enc-R")) -> ()
            n485 = global write "Robot Global Data.vi" "A Drv"(TRUE ("A Drv")) -> ()
            n486 = global write "Robot Global Data.vi" "Flywheel On"(TRUE ("A Drv")) -> ()
            n487 = global write "Robot Global Data.vi" "VX Align"(FALSE ("VX Align")) -> ()
            n488 = Wait (ms)(milliseconds to wait=u32 2000) -> ()  [unwired: 1 out]
          }
          frame #1 {
            n489 = global write "Robot Global Data.vi" "OC_Shoot"(TRUE ("A Drv")) -> ()
            n490 = Wait (ms)(milliseconds to wait=u32 1000) -> ()  [unwired: 1 out]
          }
          frame #2 {
          }
          frame #3 {
            n491 = for {
              N: 40 -> [_]
              stop <- w553 stop-if-true
              w556 = 0.3125 ("x")
              n492 = global read "Robot Global Data.vi" "V00"() -> (w555:dbl)
              n493 = global read "Robot Global Data.vi" "Drv Dist Av"() -> (w562:dbl)
              n494 = Negate(x=w555) -> (-x=w554:dbl)
              n495 = Negate(x=w556) -> (-x=w557:dbl)
              n496 = Add(x=w557, y=w554) -> (x+y=w559:dbl)
              n497 = Absolute Value(x=w562) -> (abs(x)=w561:dbl)
              n498 = Add(x=w556, y=w555) -> (x+y=w558:dbl)
              n499 = global write "Robot Global Data.vi" "A Drv-R"(w559) -> ()
              n500 = global write "Robot Global Data.vi" "A Drv-L"(w558) -> ()
              n501 = Greater Or Equal?(x=w561, y=4.0) -> (x >= y?=w553:bool)
              n502 = Wait (ms)(milliseconds to wait=u32 100) -> ()  [unwired: 1 out]
            }
          }
          frame #4 {
            n503 = global write "Robot Global Data.vi" "D_Enc-R"(TRUE ("D_Enc-R")) -> ()
            n504 = Wait (ms)(milliseconds to wait=u32 500) -> ()  [unwired: 1 out]
          }
          frame #5 {
          }
          frame #6 {
          }
          frame #7 {
          }
          frame #8 {
          }
          frame #9 {
            n505 = global write "Robot Global Data.vi" "Precision"(FALSE ("Precision")) -> ()
            n506 = global write "Robot Global Data.vi" "OC_Shoot"(FALSE ("A Drv")) -> ()
            n507 = global write "Robot Global Data.vi" "A Drv"(FALSE ("A Drv")) -> ()
            n508 = global write "Robot Global Data.vi" "Auto TS"(i8 0 ("Auto TS")) -> ()
            n509 = global write "Robot Global Data.vi" "Carriage Pos"(T1."Tee" ("Carriage Pos")) -> ()
          }
        }
      }
      frame 6 {
        n510 = flat-sequence {
          frame #0 {
            n511 = global write "Robot Global Data.vi" "Carriage Pos"(T1."High" ("Carriage Pos")) -> ()
            n512 = global write "Robot Global Data.vi" "D_Enc-R"(TRUE ("D_Enc-R")) -> ()
            n513 = global write "Robot Global Data.vi" "A Drv"(TRUE ("A Drv")) -> ()
            n514 = global write "Robot Global Data.vi" "Flywheel On"(TRUE ("A Drv")) -> ()
            n515 = global write "Robot Global Data.vi" "VX Align"(FALSE ("VX Align")) -> ()
            n516 = Wait (ms)(milliseconds to wait=u32 2000) -> ()  [unwired: 1 out]
          }
          frame #1 {
            n517 = global write "Robot Global Data.vi" "OC_Shoot"(TRUE ("A Drv")) -> ()
            n518 = Wait (ms)(milliseconds to wait=u32 1000) -> ()  [unwired: 1 out]
          }
          frame #2 {
            n519 = global write "Robot Global Data.vi" "OC_Shoot"(FALSE ("A Drv")) -> ()
            n520 = Wait (ms)(milliseconds to wait=u32 2000) -> ()  [unwired: 1 out]
          }
          frame #3 {
            n521 = global write "Robot Global Data.vi" "OC_Shoot"(TRUE ("A Drv")) -> ()
            n522 = Wait (ms)(milliseconds to wait=u32 2000) -> ()  [unwired: 1 out]
          }
          frame #4 {
            n523 = for {
              N: 40 -> [_]
              stop <- w584 stop-if-true
              w587 = 0.3125 ("x")
              n524 = global read "Robot Global Data.vi" "V00"() -> (w586:dbl)
              n525 = global read "Robot Global Data.vi" "Drv Dist Av"() -> (w593:dbl)
              n526 = Negate(x=w586) -> (-x=w585:dbl)
              n527 = Negate(x=w587) -> (-x=w588:dbl)
              n528 = Add(x=w588, y=w585) -> (x+y=w590:dbl)
              n529 = Absolute Value(x=w593) -> (abs(x)=w592:dbl)
              n530 = Add(x=w587, y=w586) -> (x+y=w589:dbl)
              n531 = global write "Robot Global Data.vi" "A Drv-R"(w590) -> ()
              n532 = global write "Robot Global Data.vi" "A Drv-L"(w589) -> ()
              n533 = Greater Or Equal?(x=w592, y=4.0) -> (x >= y?=w584:bool)
              n534 = Wait (ms)(milliseconds to wait=u32 100) -> ()  [unwired: 1 out]
            }
          }
          frame #5 {
            n535 = global write "Robot Global Data.vi" "D_Enc-R"(TRUE ("D_Enc-R")) -> ()
            n536 = Wait (ms)(milliseconds to wait=u32 500) -> ()  [unwired: 1 out]
          }
          frame #6 {
            n537 = Wait (ms)(milliseconds to wait=u32 1000) -> ()  [unwired: 1 out]
            n538 = global write "Robot Global Data.vi" "Carriage Pos"(T1."U" ("Carriage Pos")) -> ()
          }
          frame #7 {
            n539 = global write "Robot Global Data.vi" "Flywheel On"(TRUE ("A Drv")) -> ()
            n540 = global write "Robot Global Data.vi" "Precision"(FALSE ("Precision")) -> ()
            n541 = global write "Robot Global Data.vi" "OC_Shoot"(FALSE ("A Drv")) -> ()
            n542 = global write "Robot Global Data.vi" "A Drv"(FALSE ("A Drv")) -> ()
            n543 = global write "Robot Global Data.vi" "Auto TS"(i8 0 ("Auto TS")) -> ()
            n544 = global write "Robot Global Data.vi" "Carriage Pos"(T1."Cargo" ("Carriage Pos")) -> ()
          }
        }
      }
    }
    n545 = Wait (ms)(milliseconds to wait=u32 100) -> ()  [unwired: 1 out]
  }
  n546 = call <vilib>:"CTRE_Phoenix_MotorControl_RefNumRegistryGet.vi"("refnum name"="B_LA_L") -> ("PhoenixMotorControlDevRef"=w26:T15)  [unwired: 9 in, 1 out]
  n547 = call <vilib>:"CTRE_Phoenix_MotorControl_RefNumRegistryGet.vi"("refnum name"="B_LA_R") -> ("PhoenixMotorControlDevRef"=w25:T15)  [unwired: 9 in, 1 out]
  n548 = while {
    stop <- FALSE stop-if-true
    # "Tee Positioning"
    n549 = global read "Robot Global Data.vi" "Climb On"() -> (w605:bool)
    n550 = Not(x=w605) -> (.not. x?=w606:bool)
    n551 = case shown="True" w606 {
      frame False {
      }
      frame True {
        n552 = global read "Robot Global Data.vi" "Carriage Pos"() -> (w608:T1)
        n553 = case shown="\"Eject\"" w608 {
          frame "Do Nothing", Default {
          }
          frame "Cargo" {
            n554 = flat-sequence {
              frame #0 {
                n555 = global read "Robot Global Data.vi" "V11"() -> (w609:dbl)
                n556 = Add(x=w609, y=176.0 ("Desired Tee_Pot")) -> (x+y=w610:dbl)
                n557 = global write "Robot Global Data.vi" "Intake Pwr"(1.0 ("Desired Tee_Pot")) -> ()
                n558 = global write "Robot Global Data.vi" "Desired Speed"(-10000.0 ("Desired Tee_Pot")) -> ()
                n559 = global write "Robot Global Data.vi" "Desired Tee_Pot"(w610) -> ()
              }
              frame #1 {
                n560 = for {
                  N: 50 -> [_]
                  stop <- w615 stop-if-true
                  n561 = global read "Robot Global Data.vi" "Tee_Pot"() -> (w618:dbl)
                  n562 = In Range and Coerce(upper limit=259.0, x=w618, lower limit=161.0) -> (In Range?=w615:bool)  [unwired: 1 out]
                  n563 = Wait (ms)(milliseconds to wait=u32 50) -> ()  [unwired: 1 out]
                }
              }
              frame #2 {
                n564 = global write "Robot Global Data.vi" "Carriage Pos"(T2."Do Nothing" ("Carriage Pos")) -> ()
                n565 = global write "Robot Global Data.vi" "Tee-Out"(TRUE ("Tee-Out")) -> ()
              }
            }
          }
          frame "Low" {
            # "Done"
            n566 = flat-sequence {
              frame #0 {
                n567 = global write "Robot Global Data.vi" "Flywheel Power"(0.4 ("Flywheel Power")) -> ()
                n568 = global write "Robot Global Data.vi" "Fly_Adjust"(TRUE ("LED 1")) -> ()
              }
              frame #1 {
                n569 = global read "Robot Global Data.vi" "Tee-Out"() -> (w624:bool)
                n570 = case shown="True" w624 {
                  frame False {
                  }
                  frame True {
                    n571 = global write "Robot Global Data.vi" "Tee-Out"(FALSE ("Tee-Out")) -> ()
                    n572 = Wait (ms)(milliseconds to wait=u32 1500) -> ()  [unwired: 1 out]
                  }
                }
              }
              frame #2 {
                n573 = global read "Robot Global Data.vi" "V03"() -> (w627:dbl)
                n574 = Add(x=w627, y=252.0 ("Desired Tee_Pot")) -> (x+y=w628:dbl)
                n575 = global write "Robot Global Data.vi" "Desired Tee_Pot"(w628) -> ()
                n576 = Wait (ms)(milliseconds to wait=u32 1000) -> ()  [unwired: 1 out]
                n577 = global write "Robot Global Data.vi" "Intake Pwr"(0.0 ("Desired Tee_Pot")) -> ()
              }
              frame #3 {
                n578 = global read "Robot Global Data.vi" "V07"() -> (w632:dbl)
                n579 = Add(x=w632, y=8000.0 ("Desired Tee_Pot")) -> (x+y=w633:dbl)
                n580 = global write "Robot Global Data.vi" "Fly_Adjust"(FALSE ("LED 1")) -> ()
                n581 = global write "Robot Global Data.vi" "Desired Speed"(w633) -> ()
              }
              frame #4 {
                n582 = global write "Robot Global Data.vi" "Carriage Pos"(T2."Do Nothing" ("Carriage Pos")) -> ()
              }
            }
          }
          frame "High" {
            n583 = flat-sequence {
              frame #0 {
                n584 = global write "Robot Global Data.vi" "Fly_Adjust"(TRUE ("LED 1")) -> ()
                n585 = global write "Robot Global Data.vi" "Flywheel Power"(0.6 ("Flywheel Power")) -> ()
              }
              frame #1 {
                n586 = global read "Robot Global Data.vi" "Tee-Out"() -> (w639:bool)
                n587 = case shown="True" w639 {
                  frame False {
                  }
                  frame True {
                    n588 = global write "Robot Global Data.vi" "Tee-Out"(FALSE ("Tee-Out")) -> ()
                    n589 = Wait (ms)(milliseconds to wait=u32 1500) -> ()  [unwired: 1 out]
                  }
                }
              }
              frame #2 {
                n590 = global read "Robot Global Data.vi" "V04"() -> (w642:dbl)
                n591 = Add(x=241.0 ("Desired Tee_Pot"), y=w642) -> (x+y=w643:dbl)
                n592 = global write "Robot Global Data.vi" "Intake Pwr"(0.0 ("Desired Tee_Pot")) -> ()
                n593 = global write "Robot Global Data.vi" "Desired Tee_Pot"(w643) -> ()
                n594 = Wait (ms)(milliseconds to wait=u32 1200) -> ()  [unwired: 1 out]
              }
              frame #3 {
                n595 = global read "Robot Global Data.vi" "V08"() -> (w647:dbl)
                n596 = global write "Robot Global Data.vi" "Fly_Adjust"(FALSE ("LED 1")) -> ()
                n597 = Add(x=11100.0 ("Desired Tee_Pot"), y=w647) -> (x+y=w648:dbl)
                n598 = global write "Robot Global Data.vi" "Desired Speed"(w648) -> ()
              }
              frame #4 {
                n599 = global write "Robot Global Data.vi" "Carriage Pos"(T2."Do Nothing" ("Carriage Pos")) -> ()
              }
            }
          }
          frame "Long Shot" {
            n600 = flat-sequence {
              frame #0 {
                n601 = global write "Robot Global Data.vi" "Flywheel Power"(0.64 ("Flywheel Power")) -> ()
                n602 = global write "Robot Global Data.vi" "Fly_Adjust"(TRUE ("LED 1")) -> ()
              }
              frame #1 {
                n603 = global read "Robot Global Data.vi" "Tee-Out"() -> (w654:bool)
                n604 = case shown="True" w654 {
                  frame False {
                  }
                  frame True {
                    n605 = global write "Robot Global Data.vi" "Tee-Out"(FALSE ("Tee-Out")) -> ()
                    n606 = Wait (ms)(milliseconds to wait=u32 1500) -> ()  [unwired: 1 out]
                  }
                }
              }
              frame #2 {
                n607 = global read "Robot Global Data.vi" "V05"() -> (w657:dbl)
                n608 = Add(x=w657, y=247.0 ("Desired Tee_Pot")) -> (x+y=w658:dbl)
                n609 = global write "Robot Global Data.vi" "Intake Pwr"(0.0 ("Desired Tee_Pot")) -> ()
                n610 = global write "Robot Global Data.vi" "Desired Tee_Pot"(w658) -> ()
                n611 = Wait (ms)(milliseconds to wait=u32 1200) -> ()  [unwired: 1 out]
              }
              frame #3 {
                n612 = global read "Robot Global Data.vi" "V09"() -> (w662:dbl)
                n613 = Add(x=13000.0 ("Desired Tee_Pot"), y=w662) -> (x+y=w663:dbl)
                n614 = global write "Robot Global Data.vi" "Fly_Adjust"(FALSE ("LED 1")) -> ()
                n615 = global write "Robot Global Data.vi" "Desired Speed"(w663) -> ()
              }
              frame #4 {
                n616 = global write "Robot Global Data.vi" "Carriage Pos"(T2."Do Nothing" ("Carriage Pos")) -> ()
              }
            }
          }
          frame "U" {
            n617 = flat-sequence {
              frame #0 {
                n618 = global read "Robot Global Data.vi" "Tee-Out"() -> (w667:bool)
                n619 = case shown="True" w667 {
                  frame False {
                  }
                  frame True {
                    n620 = global write "Robot Global Data.vi" "Tee-Out"(FALSE ("Tee-Out")) -> ()
                    n621 = Wait (ms)(milliseconds to wait=u32 1500) -> ()  [unwired: 1 out]
                  }
                }
              }
              frame #1 {
                n622 = global write "Robot Global Data.vi" "Desired Tee_Pot"(239.0 ("Desired Tee_Pot")) -> ()
                n623 = global write "Robot Global Data.vi" "Desired Speed"(0.0 ("Desired Tee_Pot")) -> ()
                n624 = global write "Robot Global Data.vi" "Intake Pwr"(0.0 ("Desired Tee_Pot")) -> ()
              }
              frame #2 {
                n625 = global write "Robot Global Data.vi" "Carriage Pos"(T2."Do Nothing" ("Carriage Pos")) -> ()
              }
            }
          }
          frame "Hook" {
            n626 = flat-sequence {
              frame #0 {
                n627 = global read "Robot Global Data.vi" "Tee-Out"() -> (w674:bool)
                n628 = case shown="True" w674 {
                  frame False {
                  }
                  frame True {
                    n629 = global write "Robot Global Data.vi" "Tee-Out"(FALSE ("Tee-Out")) -> ()
                    n630 = Wait (ms)(milliseconds to wait=u32 1500) -> ()  [unwired: 1 out]
                  }
                }
              }
              frame #1 {
                n631 = global write "Robot Global Data.vi" "Desired Tee_Pot"(147.0 ("Desired Tee_Pot")) -> ()
                n632 = global write "Robot Global Data.vi" "Desired Speed"(0.0 ("Desired Tee_Pot")) -> ()
                n633 = global write "Robot Global Data.vi" "Intake Pwr"(0.0 ("Desired Tee_Pot")) -> ()
              }
              frame #2 {
                n634 = global write "Robot Global Data.vi" "Carriage Pos"(T2."Do Nothing" ("Carriage Pos")) -> ()
              }
            }
          }
          frame "Tee" {
            n635 = flat-sequence {
              frame #0 {
                n636 = global read "Robot Global Data.vi" "Tee-Out"() -> (w681:bool)
                n637 = case shown="True" w681 {
                  frame False {
                  }
                  frame True {
                    n638 = global write "Robot Global Data.vi" "Tee-Out"(FALSE ("Tee-Out")) -> ()
                    n639 = Wait (ms)(milliseconds to wait=u32 1500) -> ()  [unwired: 1 out]
                  }
                }
              }
              frame #1 {
                n640 = global read "Robot Global Data.vi" "V06"() -> (w684:dbl)
                n641 = Add(x=w684, y=182.0 ("Desired Tee_Pot")) -> (x+y=w685:dbl)
                n642 = global write "Robot Global Data.vi" "Desired Speed"(0.0 ("Desired Tee_Pot")) -> ()
                n643 = global write "Robot Global Data.vi" "Intake Pwr"(0.0 ("Desired Tee_Pot")) -> ()
                n644 = global write "Robot Global Data.vi" "Desired Tee_Pot"(w685) -> ()
              }
              frame #2 {
                n645 = global write "Robot Global Data.vi" "Carriage Pos"(T2."Do Nothing" ("Carriage Pos")) -> ()
              }
            }
          }
          frame "Eject" {
            n646 = flat-sequence {
              frame #0 {
                n647 = global write "Robot Global Data.vi" "Desired Speed"(9000.0 ("Desired Tee_Pot")) -> ()
                n648 = Wait (ms)(milliseconds to wait=u32 750) -> ()  [unwired: 1 out]
              }
              frame #1 {
                n649 = global read "Robot Global Data.vi" "Tee-Out"() -> (w692:bool)
                n650 = case shown="True" w692 {
                  frame False {
                  }
                  frame True {
                    n651 = global write "Robot Global Data.vi" "Tee-Out"(FALSE ("Tee-Out")) -> ()
                    n652 = Wait (ms)(milliseconds to wait=u32 500) -> ()  [unwired: 1 out]
                  }
                }
              }
              frame #2 {
                n653 = global write "Robot Global Data.vi" "Desired Tee_Pot"(182.0 ("Desired Tee_Pot")) -> ()
                n654 = Wait (ms)(milliseconds to wait=u32 750) -> ()  [unwired: 1 out]
              }
              frame #3 {
                n655 = global write "Robot Global Data.vi" "Intake Pwr"(-1.0 ("Desired Tee_Pot")) -> ()
                n656 = Wait (ms)(milliseconds to wait=u32 500) -> ()  [unwired: 1 out]
              }
              frame #4 {
                n657 = global write "Robot Global Data.vi" "Intake Pwr"(0.0 ("Desired Tee_Pot")) -> ()
                n658 = global write "Robot Global Data.vi" "Desired Speed"(0.0 ("Desired Tee_Pot")) -> ()
                n659 = global write "Robot Global Data.vi" "Carriage Pos"(T2."Do Nothing" ("Carriage Pos")) -> ()
              }
            }
          }
        }
      }
    }
    n660 = Wait (ms)(milliseconds to wait=u32 100) -> ()  [unwired: 1 out]
  }
  n661 = while {
    stop <- FALSE stop-if-true
    n662 = global read "Robot Global Data.vi" "Backup"() -> (w704:bool)
    n663 = case shown="True" w704 {
      frame False {
      }
      frame True {
        n664 = flat-sequence {
          frame #0 {
            n665 = global write "Robot Global Data.vi" "D_Enc-R"(TRUE ("D_Enc-R")) -> ()
            n666 = global write "Robot Global Data.vi" "A Drv"(TRUE ("A Drv")) -> ()
            n667 = Wait (ms)(milliseconds to wait=u32 250) -> ()  [unwired: 1 out]
          }
          frame #1 {
            n668 = for {
              N: 40 -> [_]
              stop <- w710 stop-if-true
              w713 = 0.3125 ("x")
              n669 = global read "Robot Global Data.vi" "V00"() -> (w712:dbl)
              n670 = global read "Robot Global Data.vi" "Drv Dist Av"() -> (w719:dbl)
              n671 = Negate(x=w712) -> (-x=w711:dbl)
              n672 = Negate(x=w713) -> (-x=w714:dbl)
              n673 = Add(x=w714, y=w711) -> (x+y=w716:dbl)
              n674 = Absolute Value(x=w719) -> (abs(x)=w718:dbl)
              n675 = Add(x=w713, y=w712) -> (x+y=w715:dbl)
              n676 = global write "Robot Global Data.vi" "A Drv-R"(w716) -> ()
              n677 = global write "Robot Global Data.vi" "A Drv-L"(w715) -> ()
              n678 = Greater Or Equal?(x=w718, y=1.2) -> (x >= y?=w710:bool)
              n679 = Wait (ms)(milliseconds to wait=u32 100) -> ()  [unwired: 1 out]
            }
          }
          frame #2 {
            n680 = global write "Robot Global Data.vi" "OC_Align VX"(TRUE ("A Drv")) -> ()
            n681 = global write "Robot Global Data.vi" "D_Enc-R"(TRUE ("D_Enc-R")) -> ()
            n682 = global write "Robot Global Data.vi" "A Drv"(FALSE ("A Drv")) -> ()
            n683 = global write "Robot Global Data.vi" "Backup"(FALSE ("Backup")) -> ()
            n684 = global write "Robot Global Data.vi" "A Drv-L"(0.0 ("A Drv-L")) -> ()
            n685 = global write "Robot Global Data.vi" "A Drv-R"(0.0 ("A Drv-R")) -> ()
          }
        }
      }
    }
    n686 = Wait (ms)(milliseconds to wait=u32 100) -> ()  [unwired: 1 out]
  }
  n687 = while {
    stop <- FALSE stop-if-true
    # "Vision Processing X-Axis\n[Auto Centering]"
    n688 = global read "Robot Global Data.vi" "VX Align"() -> (w727:bool)
    n689 = global read "Robot Global Data.vi" "Climb On"() -> (w729:bool)
    n690 = Not(x=w729) -> (.not. x?=w726:bool)
    n691 = Compound Arithmetic op=AND(w727, w726) -> (w728:bool)
    n692 = case shown="True" w728 {
      frame False {
      }
      frame True {
        n693 = flat-sequence {
          frame #0 {
            n694 = global write "Robot Global Data.vi" "A Drv"(TRUE ("Rumble")) -> ()
            n695 = global write "Robot Global Data.vi" "A Exit"(FALSE ("Rumble")) -> ()
            n696 = global write "Robot Global Data.vi" "Centering"(TRUE ("Centering")) -> ()
          }
          frame #1 {
            w735 = FALSE ("A Exit")
            n697 = for {
              N: 100 -> [_]
              shift-right: [w743] -> _
              shift-left: w735 -> [w742]
              shift-left: w735 -> [w741]
              shift-left: w735 -> [w740]
              shift-left: w735 -> [w739]
              stop <- w752 stop-if-true
              w745 = 0.2 ("y")
              w753 = -35.0 ("y")
              w754 = 35.0 ("y")
              w760 = -400.0 ("y")
              w761 = 400.0 ("y")
              # "To check if past four\niterations of loop has\nA Exit true; Aprrox.\nCentered"
              n698 = global read "Robot Global Data.vi" "Lime X"() -> (w737:dbl)
              n699 = global read "Robot Global Data.vi" "Drv Input 1"() -> (w748:dbl)
              n700 = global read "Robot Global Data.vi" "Drv Input 2"() -> (w750:dbl)
              n701 = Wait (ms)(milliseconds to wait=u32 100) -> ()  [unwired: 1 out]
              n702 = Compound Arithmetic op=AND(w742, w741, w740, w739) -> (w738:bool)
              n703 = Absolute Value(x=w748) -> (abs(x)=w749:dbl)
              n704 = Absolute Value(x=w750) -> (abs(x)=w751:dbl)
              n705 = Greater?(x=w749, y=w745) -> (0:w746:bool)
              n706 = Greater?(x=w751, y=w745) -> (0:w747:bool)
              n707 = In Range and Coerce(upper limit=1000.0, x=w737, lower limit=w761) -> (In Range?=w757:bool)  [unwired: 1 out]
              n708 = In Range and Coerce(upper limit=w761, x=w737, lower limit=w754) -> (In Range?=w758:bool)  [unwired: 1 out]
              n709 = In Range and Coerce(upper limit=w754, x=w737, lower limit=w753) -> (In Range?=w759:bool)  [unwired: 1 out]
              n710 = In Range and Coerce(upper limit=w753, x=w737, lower limit=w760) -> (In Range?=w756:bool)  [unwired: 1 out]
              n711 = In Range and Coerce(upper limit=w760, x=w737, lower limit=-1000.0) -> (In Range?=w755:bool)  [unwired: 1 out]
              n712 = Or(x=w746, y=w747) -> (x .or. y?=w744:bool)
              n713 = case shown="True" w756 {
                frame False {
                }
                frame True {
                  n714 = global read "Robot Global Data.vi" "V10"() -> (w770:dbl)
                  n715 = Subtract(x=-0.075 ("4Bar Auto"), y=w770) -> (x-y=w768:dbl)
                  n716 = global write "Robot Global Data.vi" "A Drv-L"(w768) -> ()
                  n717 = global write "Robot Global Data.vi" "A Drv-R"(w768) -> ()
                }
              }
              n718 = case shown="True" w757 {
                frame False {
                }
                frame True {
                  n719 = global read "Robot Global Data.vi" "V01"() -> (w778:dbl)
                  n720 = Add(x=0.2 ("4Bar Auto"), y=w778) -> (x+y=w776:dbl)
                  n721 = global write "Robot Global Data.vi" "A Drv-L"(w776) -> ()
                  n722 = global write "Robot Global Data.vi" "A Drv-R"(w776) -> ()
                }
              }
              n723 = case shown="True" w758 {
                frame False {
                }
                frame True {
                  n724 = global read "Robot Global Data.vi" "V10"() -> (w775:dbl)
                  n725 = Add(x=0.075 ("4Bar Auto"), y=w775) -> (x+y=w773:dbl)
                  n726 = global write "Robot Global Data.vi" "A Drv-L"(w773) -> ()
                  n727 = global write "Robot Global Data.vi" "A Drv-R"(w773) -> ()
                }
              }
              n728 = case shown="True" w759 {
                frame False {
                }
                frame True {
                  w771 = 0.0 ("4Bar Auto")
                  n729 = global write "Robot Global Data.vi" "A Drv-L"(w771) -> ()
                  n730 = global write "Robot Global Data.vi" "A Drv-R"(w771) -> ()
                  n731 = global write "Robot Global Data.vi" "A Exit"(TRUE ("A Exit")) -> ()
                }
              }
              n732 = case shown="True" w755 {
                frame False {
                }
                frame True {
                  n733 = global read "Robot Global Data.vi" "V01"() -> (w767:dbl)
                  n734 = Subtract(x=-0.2 ("4Bar Auto"), y=w767) -> (x-y=w765:dbl)
                  n735 = global write "Robot Global Data.vi" "A Drv-L"(w765) -> ()
                  n736 = global write "Robot Global Data.vi" "A Drv-R"(w765) -> ()
                }
              }
              n737 = global read "Robot Global Data.vi" "A Exit"() -> (w743:bool)
              n738 = Or(x=w738, y=w744) -> (x .or. y?=w752:bool)
            }
          }
          frame #2 {
            n739 = global write "Robot Global Data.vi" "A Drv"(FALSE ("Rumble")) -> ()
            n740 = global write "Robot Global Data.vi" "A Exit"(FALSE ("Rumble")) -> ()
            n741 = global write "Robot Global Data.vi" "VX Align"(FALSE ("VX Align")) -> ()
            n742 = global write "Robot Global Data.vi" "Centering"(FALSE ("Centering")) -> ()
          }
        }
      }
    }
    n743 = Wait (ms)(milliseconds to wait=u32 100) -> ()  [unwired: 1 out]
  }
  n744 = while {
    tunnel: w26 -> [w847]
    tunnel: w25 -> [w846]
    tunnel: [w850] -> _
    tunnel: [w849] -> _
    stop <- FALSE stop-if-true
    w848 = T19 0 items=["PercentOutput"=0, "Position"=1, "Velocity"=2, "Current"=3, "Follower"=5, "MotionProfile"=6, "MotionMagic"=7, "MotionProfileArc"=10, "Disabled"=15] ("Control Mode")
    # "Adjust Robot Pull Up Speed\nDon't worry about:\nNo Load Raise Arms and\nDrop Down Speeds"
    # "Upper & Lower Thresholds"
    # "Trailing Bar Driver"
    # "*May need to negate Linear Actuator\npower due to motor configuration"
    n745 = global read "Robot Global Data.vi" "OC_LA_Reset"() -> (w845:bool)
    n746 = global read "Robot Global Data.vi" "Climb On"() -> (w836:bool)
    n747 = global read "Robot Global Data.vi" "TB Power"() -> (w786:dbl)
    n748 = case shown="True" w845 {
      tunnel: w847 -> [w882 w888]
      tunnel: w846 -> [w881 w887]
      tunnel: [w882 w885] -> w844
      tunnel: [w881 w883] -> w843
      frame False {
      }
      frame True {
        n749 = flat-sequence {
          tunnel: w888 -> [w891]
          tunnel: w887 -> [w892]
          tunnel: [w890] -> w886
          tunnel: [w889] -> w884
          tunnel: [w896] -> w885
          tunnel: w886 -> [w896]
          tunnel: [w895] -> w883
          tunnel: w884 -> [w895]
          frame #0 {
            n750 = call <vilib>:"CTRE_Phoenix_MotorControl_SetSelectedSensorPosition.vi"("New Sensor Position"=0, "PhoenixMotorControlDevRef"=w892) -> ("PhoenixMotorControlDevRef"=w889:T15)  [unwired: 8 in, 1 out]
            n751 = call <vilib>:"CTRE_Phoenix_MotorControl_SetSelectedSensorPosition.vi"("New Sensor Position"=0, "PhoenixMotorControlDevRef"=w891) -> ("PhoenixMotorControlDevRef"=w890:T15)  [unwired: 8 in, 1 out]
          }
          frame #1 {
            n752 = global write "Robot Global Data.vi" "OC_LA_Reset"(FALSE ("OC_LA_Reset")) -> ()
          }
        }
      }
    }
    n753 = Select(t=w786, s=w836, f=0.0) -> (s? t:f=w808:dbl)
    n754 = global read "Robot Global Data.vi" "TBar L"() -> (w830:dbl)
    n755 = global read "Robot Global Data.vi" "TBar R"() -> (w818:dbl)
    n756 = In Range and Coerce(upper limit=1.0, x=w808, lower limit=0.0) -> (coerced(x)=w832:dbl)  [unwired: 1 out]
    n757 = In Range and Coerce(upper limit=1.0, x=w808, lower limit=0.0) -> (coerced(x)=w820:dbl)  [unwired: 1 out]
    n758 = Less?(x=w830, y=10.0) -> (x < y?=w829:bool)
    n759 = Less?(x=w818, y=10.0) -> (x < y?=w817:bool)
    n760 = Select(t=w832, s=w829, f=w808) -> (s? t:f=w823:dbl)
    n761 = Select(t=w820, s=w817, f=w808) -> (s? t:f=w811:dbl)
    n762 = global read "Robot Global Data.vi" "TBar L"() -> (w825:dbl)
    n763 = global read "Robot Global Data.vi" "TBar R"() -> (w813:dbl)
    n764 = call-poly <vilib>:"CTRE_Phoenix_MotorController_Get_Enhanced.vi"("PhoenixMotorControlDevRef"=w844) -> ("PhoenixMotorControlDevRef"=w841:T15, "Quadrature Position"=w842:i32)  [unwired: 11 in, 2 out]
    n765 = call-poly <vilib>:"CTRE_Phoenix_MotorController_Get_Enhanced.vi"("PhoenixMotorControlDevRef"=w843) -> ("PhoenixMotorControlDevRef"=w840:T15, "Quadrature Position"=w838:i32)  [unwired: 11 in, 2 out]
    n766 = In Range and Coerce(upper limit=0.0, x=w823, lower limit=-1.0) -> (coerced(x)=w826:dbl)  [unwired: 1 out]
    n767 = In Range and Coerce(upper limit=0.0, x=w811, lower limit=-1.0) -> (coerced(x)=w814:dbl)  [unwired: 1 out]
    n768 = Greater?(x=w825, y=91.0) -> (0:w824:bool)
    n769 = Greater?(x=w813, y=95.0) -> (0:w812:bool)
    n770 = Select(t=w826, s=w824, f=w823) -> (s? t:f=w791:dbl)
    n771 = Select(t=w814, s=w812, f=w811) -> (s? t:f=w810:dbl)
    n772 = Multiply(x=w786, y=0.5) -> (x*y=w794:dbl)
    n773 = Multiply(x=w791, y=1.0) -> (x*y=w790:dbl)
    n774 = Multiply(x=w810, y=1.0) -> (x*y=w789:dbl)
    n775 = Divide(x=w842, y=-2632) -> (x/y=w807:dbl)
    n776 = Divide(x=w838, y=2643) -> (x/y=w803:dbl)
    n777 = global read "Robot Global Data.vi" "TB Power"() -> (w783:dbl)
    n778 = Multiply(x=w807, y=1.42) -> (x*y=w805:dbl)
    n779 = Multiply(x=w803, y=1.42) -> (x*y=w802:dbl)
    n780 = Greater?(x=w783, y=0.0) -> (0:w784:bool)
    n781 = case shown="True" w784 {
      tunnel: w790 -> [w856 w869]
      tunnel: w789 -> [w855 w870]
      tunnel: [w854 w868] -> w788
      tunnel: [w853 w867] -> w787
      frame False {
        # "Right"
        # "Left"
        # "Down"
        n782 = global read "Robot Global Data.vi" "TBar R"() -> (w865:dbl)
        n783 = global read "Robot Global Data.vi" "TBar R"() -> (w860:dbl)
        n784 = global read "Robot Global Data.vi" "TBar L"() -> (w866:dbl)
        n785 = global read "Robot Global Data.vi" "TBar L"() -> (w859:dbl)
        n786 = Less?(x=w866, y=w865) -> (x < y?=w864:bool)
        n787 = Less?(x=w860, y=w859) -> (x < y?=w862:bool)
        n788 = Multiply(x=w856, y=0.9) -> (x*y=w863:dbl)
        n789 = Multiply(x=w855, y=0.9) -> (x*y=w861:dbl)
        n790 = Select(t=w863, s=w864, f=w856) -> (s? t:f=w854:dbl)
        n791 = Select(t=w861, s=w862, f=w855) -> (s? t:f=w853:dbl)
      }
      frame True {
        # "Right"
        # "Left"
        # "Up"
        n792 = global read "Robot Global Data.vi" "TBar R"() -> (w879:dbl)
        n793 = global read "Robot Global Data.vi" "TBar R"() -> (w874:dbl)
        n794 = global read "Robot Global Data.vi" "TBar L"() -> (w880:dbl)
        n795 = global read "Robot Global Data.vi" "TBar L"() -> (w873:dbl)
        n796 = Greater?(x=w880, y=w879) -> (0:w878:bool)
        n797 = Greater?(x=w874, y=w873) -> (0:w877:bool)
        n798 = Multiply(x=w869, y=0.8) -> (x*y=w876:dbl)
        n799 = Multiply(x=w870, y=0.8) -> (x*y=w875:dbl)
        n800 = Select(t=w876, s=w878, f=w869) -> (s? t:f=w868:dbl)
        n801 = Select(t=w875, s=w877, f=w870) -> (s? t:f=w867:dbl)
      }
    }
    n802 = global write "Robot Global Data.vi" "TBar L"(w805) -> ()
    n803 = global write "Robot Global Data.vi" "TBar R"(w802) -> ()
    n804 = global read "Robot Global Data.vi" "OC_ TB Override"() -> (w796:bool)
    n805 = Negate(x=w794) -> (-x=w798:dbl)
    n806 = Negate(x=w788) -> (-x=w792:dbl)
    n807 = Select(t=w794, s=w796, f=w787) -> (s? t:f=w795:dbl)
    n808 = Select(t=w798, s=w796, f=w792) -> (s? t:f=w793:dbl)
    n809 = call <vilib>:"CTRE_Phoenix_MotorControl_Set.vi"("Output"=w793, "Control Mode"=w848, "PhoenixMotorControlDevRef"=w841) -> ("PhoenixMotorControlDevRef"=w850:T15)  [unwired: 7 in, 1 out]
    n810 = call <vilib>:"CTRE_Phoenix_MotorControl_Set.vi"("Output"=w795, "Control Mode"=w848, "PhoenixMotorControlDevRef"=w840) -> ("PhoenixMotorControlDevRef"=w849:T15)  [unwired: 7 in, 1 out]
    n811 = Wait (ms)(milliseconds to wait=u32 50) -> ()  [unwired: 1 out]
  }
  n812 = while {
    tunnel: w4 -> [w941]
    tunnel: w3 -> [w940]
    tunnel: [w944] -> _
    tunnel: [w943] -> _
    stop <- FALSE stop-if-true
    w942 = T19 0 items=["PercentOutput"=0, "Position"=1, "Velocity"=2, "Current"=3, "Follower"=5, "MotionProfile"=6, "MotionMagic"=7, "MotionProfileArc"=10, "Disabled"=15] ("Control Mode")
    # "*Changed the limit switch values since it was backwards-"
    # "Rotational Thresholds"
    # "Tee/Carriage Driver"
    n813 = global read "Robot Global Data.vi" "OC_LA_Reset"() -> (w939:bool)
    n814 = global read "Robot Global Data.vi" "OC_Tee Pwr"() -> (w908:dbl)
    n815 = global read "Robot Global Data.vi" "DC Tee Pwr"() -> (w909:dbl)
    n816 = Absolute Value(x=w909) -> (abs(x)=w912:dbl)
    n817 = case shown="True" w939 {
      tunnel: w941 -> [w947 w953]
      tunnel: w940 -> [w946 w952]
      tunnel: [w947 w950] -> w938
      tunnel: [w946 w948] -> w937
      frame False {
      }
      frame True {
        n818 = flat-sequence {
          tunnel: w953 -> [w956]
          tunnel: w952 -> [w957]
          tunnel: [w955] -> w951
          tunnel: [w954] -> w949
          tunnel: [w961] -> w950
          tunnel: w951 -> [w961]
          tunnel: [w960] -> w948
          tunnel: w949 -> [w960]
          frame #0 {
            n819 = call <vilib>:"CTRE_Phoenix_MotorControl_SetSelectedSensorPosition.vi"("New Sensor Position"=0, "PhoenixMotorControlDevRef"=w957) -> ("PhoenixMotorControlDevRef"=w954:T15)  [unwired: 8 in, 1 out]
            n820 = call <vilib>:"CTRE_Phoenix_MotorControl_SetSelectedSensorPosition.vi"("New Sensor Position"=0, "PhoenixMotorControlDevRef"=w956) -> ("PhoenixMotorControlDevRef"=w955:T15)  [unwired: 8 in, 1 out]
          }
          frame #1 {
            n821 = global write "Robot Global Data.vi" "OC_LA_Reset"(FALSE ("OC_LA_Reset")) -> ()
          }
        }
      }
    }
    n822 = Greater?(x=w912, y=0.2) -> (0:w910:bool)
    n823 = Select(t=w909, s=w910, f=w908) -> (s? t:f=w904:dbl)
    n824 = Absolute Value(x=w904) -> (abs(x)=w907:dbl)
    n825 = Greater?(x=w907, y=0.2) -> (0:w905:bool)
    n826 = global read "Robot Global Data.vi" "Auto Tee Pwr"() -> (w902:dbl)
    n827 = global read "Robot Global Data.vi" "Climb On"() -> (w901:bool)
    n828 = Select(t=w904, s=w905, f=0.0) -> (s? t:f=w900:dbl)
    n829 = Select(t=w900, s=w901, f=w902) -> (s? t:f=w899:dbl)
    n830 = call-poly <vilib>:"CTRE_Phoenix_MotorController_Get_Enhanced.vi"("PhoenixMotorControlDevRef"=w938) -> ("PhoenixMotorControlDevRef"=w936:T15)  [unwired: 11 in, 3 out]
    n831 = call-poly <vilib>:"CTRE_Phoenix_MotorController_Get_Enhanced.vi"("PhoenixMotorControlDevRef"=w937) -> ("PhoenixMotorControlDevRef"=w935:T15)  [unwired: 11 in, 3 out]
    n832 = Negate(x=w899) -> (-x=w915:dbl)
    n833 = global read "Robot Global Data.vi" "Tee_Pot"() -> (w930:dbl)
    n834 = global read "Robot Global Data.vi" "Lo LS"() -> (w920:bool)
    n835 = Greater?(x=w930, y=280.0) -> (0:w919:bool)
    n836 = In Range and Coerce(upper limit=1.0, x=w915, lower limit=0.0) -> (coerced(x)=w932:dbl)  [unwired: 1 out]
    n837 = Or(x=w920, y=w919) -> (x .or. y?=w918:bool)
    n838 = Select(t=w932, s=w918, f=w915) -> (s? t:f=w924:dbl)
    n839 = global read "Robot Global Data.vi" "Tee_Pot"() -> (w925:dbl)
    n840 = global read "Robot Global Data.vi" "Hi LS"() -> (w921:bool)
    n841 = Less?(x=w925, y=80.0) -> (x < y?=w923:bool)
    n842 = In Range and Coerce(upper limit=0.0, x=w924, lower limit=-1.0) -> (coerced(x)=w927:dbl)  [unwired: 1 out]
    n843 = Or(x=w921, y=w923) -> (x .or. y?=w922:bool)
    n844 = Select(t=w927, s=w922, f=w924) -> (s? t:f=w917:dbl)
    n845 = Multiply(x=w917, y=0.55) -> (x*y=w913:dbl)
    n846 = Negate(x=w913) -> (-x=w914:dbl)
    n847 = call <vilib>:"CTRE_Phoenix_MotorControl_Set.vi"("Output"=w913, "Control Mode"=w942, "PhoenixMotorControlDevRef"=w936) -> ("PhoenixMotorControlDevRef"=w944:T15)  [unwired: 7 in, 1 out]
    n848 = call <vilib>:"CTRE_Phoenix_MotorControl_Set.vi"("Output"=w914, "Control Mode"=w942, "PhoenixMotorControlDevRef"=w935) -> ("PhoenixMotorControlDevRef"=w943:T15)  [unwired: 7 in, 1 out]
    n849 = Wait (ms)(milliseconds to wait=u32 100) -> ()  [unwired: 1 out]
  }
  n850 = while {
    stop <- FALSE stop-if-true
    # "camMode:\n     0 = Vision Processor\n     1 = Camera Only\n\nledMode:\n     0 = Mode set in pipe\n     1 = Force Off\n     2 = Force Blink\n     3 = Force On\n\ntv:\n     0 = No Target\n     1 = Target in View\n\ntx:\n     Center X Value\n\nVP Select\n      Limelight or Dash VP\n\nVP X:\n      Lime or Dash  X Center\n\nVP In View\n      Lime or Dash Target in View"
    # "Vision Processing"
    n851 = global read "Robot Global Data.vi" "CamMode"() -> (w968:i8)
    n852 = call-poly <vilib>:"NT Read Value.vi"("Name"="/limelight/tx") -> ("Numeric"=w975:dbl)  [unwired: 9 in, 1 out]
    n853 = call-poly <vilib>:"NT Read Value.vi"("Default Value"=0.0, "Name"="/limelight/tv") -> ("Numeric"=w978:dbl)  [unwired: 8 in, 1 out]
    n854 = call-poly <vilib>:"NT Read Value.vi"("Name"="/limelight/ty") -> ("Numeric"=w963:dbl)  [unwired: 9 in, 1 out]
    n855 = Equal?(x=w978, y=1.0) -> (x = y?=w976:bool)
    n856 = Multiply(x=w975, y=34.0) -> (x*y=w973:dbl)
    n857 = Multiply(x=w963, y=41.0) -> (x*y=w964:dbl)
    n858 = call-poly <vilib>:"NT Write Value.vi"("Numeric"=w968, "Name"="/limelight/camMode") -> ()  [unwired: 9 in, 1 out]
    n859 = global write "Robot Global Data.vi" "Lime In View"(w976) -> ()
    n860 = global write "Robot Global Data.vi" "Lime X"(w973) -> ()
    n861 = global write "Robot Global Data.vi" "Lime Y"(w964) -> ()
    n862 = global write "Robot Global Data.vi" "Lime Y Angle"(w963) -> ()
    n863 = global read "Robot Global Data.vi" "Lime Cam"() -> (w969:bool)
    n864 = Select(t=i8 1, s=w969, f=i8 0) -> (s? t:f=w972:i8)
    n865 = global write "Robot Global Data.vi" "CamMode"(w972) -> ()
    n866 = Wait (ms)(milliseconds to wait=u32 50) -> ()  [unwired: 1 out]
  }
  n867 = while {
    stop <- FALSE stop-if-true
    # "Read from Dashboard"
    n868 = call-poly <vilib>:"NT Read Value.vi"("Name"="D_W V-Array") -> ("Numeric Array"=w1014:dbl[])  [unwired: 9 in, 1 out]
    n869 = call-poly <vilib>:"NT Read Value.vi"("Name"="D_W String Array") -> ("String Array"=w999:string[])  [unwired: 9 in, 1 out]
    n870 = call-poly <vilib>:"NT Read Value.vi"("Name"="D_W Boolean Array") -> ("Boolean Array"=w993:bool[])  [unwired: 9 in, 1 out]
    n871 = Index Array(array=w1014) -> (element #1=w1013:dbl, element #2=w1012:dbl, element #3=w1011:dbl, element #4=w1010:dbl, element #5=w1009:dbl, element #6=w1008:dbl, element #7=w1007:dbl, element #8=w1006:dbl, element #9=w1005:dbl, element #10=w1004:dbl, element #11=w1003:dbl, element #12=w1002:dbl)  [unwired: 12 in]
    n872 = Index Array(array=w999) -> (element #1=w998:string, element #2=w997:string)  [unwired: 2 in]
    n873 = Index Array(array=w993) -> (element=w992:bool)  [unwired: 1 in]
    n874 = global write "Robot Global Data.vi" "V00"(w1013) -> ()
    n875 = global write "Robot Global Data.vi" "V01"(w1012) -> ()
    n876 = global write "Robot Global Data.vi" "V02"(w1011) -> ()
    n877 = global write "Robot Global Data.vi" "V03"(w1010) -> ()
    n878 = global write "Robot Global Data.vi" "V04"(w1009) -> ()
    n879 = global write "Robot Global Data.vi" "V05"(w1008) -> ()
    n880 = global write "Robot Global Data.vi" "V06"(w1007) -> ()
    n881 = global write "Robot Global Data.vi" "V07"(w1006) -> ()
    n882 = global write "Robot Global Data.vi" "V08"(w1005) -> ()
    n883 = global write "Robot Global Data.vi" "V09"(w1004) -> ()
    n884 = global write "Robot Global Data.vi" "V10"(w1003) -> ()
    n885 = global write "Robot Global Data.vi" "V11"(w1002) -> ()
    n886 = global write "Robot Global Data.vi" "D_Controller"(w998) -> ()
    n887 = global write "Robot Global Data.vi" "O_Controller"(w997) -> ()
    n888 = global write "Robot Global Data.vi" "OC_Change Lights"(w992) -> ()
    n889 = call-poly <vilib>:"NT Read Value.vi"("Name"="D_W Numeric Array") -> ("Numeric Array"=w996:dbl[])  [unwired: 9 in, 1 out]
    n890 = Index Array(array=w996) -> (element #1=w991:dbl, element #2=w990:dbl, element #3=w989:dbl, element #4=w988:dbl, element #5=w984:dbl, element #6=w985:dbl, element #7=w986:dbl, element #8=w987:dbl)  [unwired: 8 in]
    n891 = global write "Robot Global Data.vi" "Cam Mode"(w988) -> ()
    n892 = global write "Robot Global Data.vi" "Dash Select"(w991) -> ()
    n893 = global write "Robot Global Data.vi" "Light Select"(w990) -> ()
    n894 = global write "Robot Global Data.vi" "Key Enum"(w989) -> ()
    n895 = global write "Robot Global Data.vi" "LED Mode"(w984) -> ()
    n896 = global write "Robot Global Data.vi" "D Set Lights"(w985) -> ()
    n897 = global write "Robot Global Data.vi" "Desired Dist"(w986) -> ()
    n898 = global write "Robot Global Data.vi" "Auto Type"(w987) -> ()
    n899 = Wait (ms)(milliseconds to wait=u32 50) -> ()  [unwired: 1 out]
  }
  n900 = disable-structure shown="Disabled" {
    frame Disabled {
      n901 = call <vilib>:"WPI_JoystickRefNum Registry Get.vi"("refnum name"="Joystick 0") -> ("JoystickDevRef"=w1019:T13)  [unwired: 1 in, 9 out]
      n902 = call <vilib>:"WPI_RobotDriveRefNum Registry Get.vi"("refnum name"="Left and Right Motors") -> ("RobotDriveDevRef"=w1018:T20)  [unwired: 1 in, 9 out]
      n903 = Bundle("JoystickDevRef"=w1019, "RobotDriveDevRef"=w1018) -> (w1017:T21)  [unwired: 1 out]
      n904 = while {
        shift-right: [w1025] -> _
        shift-left: w1017 -> [w1025]
        stop <- FALSE stop-if-true
        # "10 ms tasks go here"
        n905 = Wait (ms)(milliseconds to wait=u32 10) -> ()  [unwired: 1 out]
      }
      n906 = while {
        shift-right: [w1022] -> _
        shift-left: w1017 -> [w1022]
        stop <- FALSE stop-if-true
        # "100 ms tasks go here"
        n907 = Wait (ms)(milliseconds to wait=u32 100) -> ()  [unwired: 1 out]
      }
    }
    frame Enabled {
    }
  }
  n908 = while {
    tunnel: w27 -> [w1040]
    tunnel: [w1039] -> _
    stop <- FALSE stop-if-true
    w1041 = T19 0 items=["PercentOutput"=0, "Position"=1, "Velocity"=2, "Current"=3, "Follower"=5, "MotionProfile"=6, "MotionMagic"=7, "MotionProfileArc"=10, "Disabled"=15] ("Control Mode")
    # "Carriage Belt Driver"
    n909 = global read "Robot Global Data.vi" "DC_Shoot"() -> (w1034:bool)
    n910 = global read "Robot Global Data.vi" "OC_Shoot"() -> (w1035:bool)
    n911 = global read "Robot Global Data.vi" "Intake Pwr"() -> (w1033:dbl)
    n912 = Or(x=w1034, y=w1035) -> (x .or. y?=w1032:bool)
    n913 = global read "Robot Global Data.vi" "OC_ Flywheel Off"() -> (w1036:bool)
    n914 = Select(t=-1.0, s=w1032, f=w1033) -> (s? t:f=w1029:dbl)
    n915 = Not(x=w1036) -> (.not. x?=w1037:bool)
    n916 = Select(t=w1029, s=w1037, f=0.0) -> (s? t:f=w1028:dbl)
    n917 = call <vilib>:"CTRE_Phoenix_MotorControl_Set.vi"("Output"=w1028, "Control Mode"=w1041, "PhoenixMotorControlDevRef"=w1040) -> ("PhoenixMotorControlDevRef"=w1039:T15)  [unwired: 7 in, 1 out]
    n918 = Wait (ms)(milliseconds to wait=u32 100) -> ()  [unwired: 1 out]
  }
  n919 = call <vilib>:"WPI_MotorControlRefNum Registry Get.vi"("refnum name"="B_Lights") -> ("MotorControlDevRef"=w19:T15)  [unwired: 9 in, 1 out]
  n920 = call <vilib>:"WPI_DigitalOutputRefNum Registry Get.vi"("refnum name"="B_Arduino") -> ("DigitalOutputDevRef"=w5:T22)  [unwired: 9 in, 1 out]
  n921 = while {
    stop <- FALSE stop-if-true
    # "Rumble at 40 Secs Left in Match"
    n922 = global read "Robot Global Data.vi" "Tele Time"() -> (w1044:dbl)
    n923 = In Range and Coerce(upper limit=95.5, x=w1044, lower limit=95.0) -> (In Range?=w1043:bool)  [unwired: 1 out]
    n924 = case shown="True" w1043 {
      frame False {
      }
      frame True {
        n925 = flat-sequence {
          frame #0 {
            n926 = global write "Robot Global Data.vi" "Rumble"(TRUE ("Rumble")) -> ()
            n927 = Wait (ms)(milliseconds to wait=u32 1000) -> ()  [unwired: 1 out]
          }
          frame #1 {
            n928 = global write "Robot Global Data.vi" "Rumble"(FALSE ("Rumble")) -> ()
          }
        }
      }
    }
    n929 = Wait (ms)(milliseconds to wait=u32 200) -> ()  [unwired: 1 out]
  }
  n930 = while {
    tunnel: w19 -> [w1053]
    tunnel: [w1052] -> _
    stop <- FALSE stop-if-true
    # "Robot Lights (PWM 9)"
    n931 = global read "Robot Global Data.vi" "Robot Lights"() -> (w1056:i8)
    n932 = Multiply(x=w1056, y=0.0625 ("PWM Divide")) -> (x*y=w1055:dbl)
    n933 = Subtract(x=w1055, y=1.0) -> (x-y=w1057:dbl)
    n934 = call <vilib>:"WPI_MotorControlSetOutput.vi"("Output"=w1057, "MotorControlDevRef"=w1053) -> ("MotorControlDevRef"=w1052:T15)  [unwired: 7 in, 2 out]
    n935 = Wait (ms)(milliseconds to wait=u32 200) -> ()  [unwired: 1 out]
  }
  n936 = while {
    tunnel: [w1063] -> _
    tunnel: w5 -> [w1061]
    stop <- FALSE stop-if-true
    # "Lets Arduino know we're Enabled"
    n937 = global read "Robot Global Data.vi" "Arduino"() -> (w1062:bool)
    n938 = call <vilib>:"WPI_DigitalOutputSetValue.vi"("Value"=w1062, "DigitalOutputDevRef"=w1061) -> ("DigitalOutputDevRef"=w1063:T22)  [unwired: 8 in, 1 out]
    n939 = Wait (ms)(milliseconds to wait=u32 100) -> ()  [unwired: 1 out]
  }
  n940 = while {
    stop <- FALSE stop-if-true
    # "Change Robot Lights\nfrom Dashboard"
    n941 = global read "Robot Global Data.vi" "D Set Lights"() -> (w1070:i8)
    n942 = global read "Robot Global Data.vi" "Change Lights"() -> (w1071:bool)
    n943 = global read "Robot Global Data.vi" "Robot Lights"() -> (w1069:i8)
    n944 = Select(t=w1070, s=w1071, f=w1069) -> (s? t:f=w1068:i8)
    n945 = global write "Robot Global Data.vi" "Robot Lights"(w1068) -> ()
    n946 = Wait (ms)(milliseconds to wait=u32 100) -> ()  [unwired: 1 out]
  }
  n947 = call <vilib>:"CTRE_Phoenix_MotorControl_RefNumRegistryGet.vi"("refnum name"="B_Flywheel") -> ("PhoenixMotorControlDevRef"=w30:T15)  [unwired: 9 in, 1 out]
  n948 = while {
    tunnel: w30 -> [w1085]
    tunnel: [w1083] -> _
    stop <- FALSE stop-if-true
    w1082 = T19 0 items=["PercentOutput"=0, "Position"=1, "Velocity"=2, "Current"=3, "Follower"=5, "MotionProfile"=6, "MotionMagic"=7, "MotionProfileArc"=10, "Disabled"=15] ("Control Mode")
    # "Carriage Flywheel Driver"
    n949 = global read "Robot Global Data.vi" "Flywheel On"() -> (w1077:bool)
    n950 = global read "Robot Global Data.vi" "Climb On"() -> (w1075:bool)
    n951 = global read "Robot Global Data.vi" "Flywheel Power"() -> (w1073:dbl)
    n952 = Not(x=w1075) -> (.not. x?=w1076:bool)
    n953 = And(x=w1077, y=w1076) -> (x .and. y?=w1074:bool)
    n954 = call-poly <vilib>:"CTRE_Phoenix_MotorController_Get_TalonFX.vi"("PhoenixMotorControlDevRef"=w1085) -> ("Velocity"=w1084:dbl)  [unwired: 10 in, 4 out]
    n955 = Select(t=w1073, s=w1074, f=0.0 ("t")) -> (s? t:f=w1081:dbl)
    n956 = global write "Robot Global Data.vi" "Flywheel Speed"(w1084) -> ()
    n957 = In Range and Coerce(upper limit=1.0, x=w1081, lower limit=-1.0) -> (coerced(x)=w1078:dbl)  [unwired: 1 out]
    n958 = call <vilib>:"CTRE_Phoenix_MotorControl_Set.vi"("Output"=w1078, "Control Mode"=w1082, "PhoenixMotorControlDevRef"=w1085) -> ("PhoenixMotorControlDevRef"=w1083:T15)  [unwired: 7 in, 1 out]
    n959 = Wait (ms)(milliseconds to wait=u32 100) -> ()  [unwired: 1 out]
  }
  n960 = while {
    stop <- FALSE stop-if-true
    # "FMS Color Select"
    n961 = global read "Robot Global Data.vi" "Robot Lights"() -> (w1091:i8)
    n962 = global read "Robot Global Data.vi" "Tele Time"() -> (w1095:dbl)
    n963 = call <vilib>:"WPI_DriverStationGet Alliance Info.vi"() -> ("Alliance"=w1100:T23)  [unwired: 6 in, 5 out]
    n964 = Equal?(x=w1100, y=WPI_DriverStationAllianceInfo."Blue" ("Alliance")) -> (x = y?=w1098:bool)
    n965 = Less?(x=w1095, y=1.0) -> (x < y?=w1093:bool)
    n966 = Select(t=i8 0, s=w1098, f=i8 1 ("t")) -> (s? t:f=w1092:i8)
    n967 = Select(t=w1092, s=w1093, f=w1091) -> (s? t:f=w1090:i8)
    n968 = global write "Robot Global Data.vi" "Robot Lights"(w1090) -> ()
    n969 = Wait (ms)(milliseconds to wait=u32 100) -> ()  [unwired: 1 out]
  }
  n970 = while {
    stop <- FALSE stop-if-true
    # "Climb Robot Lights\nRainbow"
    n971 = global read "Robot Global Data.vi" "Tele Time"() -> (w1108:dbl)
    n972 = global read "Robot Global Data.vi" "Robot Lights"() -> (w1105:i8)
    n973 = Greater?(x=w1108, y=105.0) -> (0:w1106:bool)
    n974 = Select(t=i8 20, s=w1106, f=w1105) -> (s? t:f=w1104:i8)
    n975 = global write "Robot Global Data.vi" "Robot Lights"(w1104) -> ()
    n976 = Wait (ms)(milliseconds to wait=u32 100) -> ()  [unwired: 1 out]
  }
  n977 = while {
    stop <- FALSE stop-if-true
    # "Pre-Climb Robot Lights\nTurquoise"
    n978 = global read "Robot Global Data.vi" "Tele Time"() -> (w1116:dbl)
    n979 = global read "Robot Global Data.vi" "Robot Lights"() -> (w1112:i8)
    n980 = In Range and Coerce(upper limit=105.0, x=w1116, lower limit=95.0) -> (In Range?=w1113:bool)  [unwired: 1 out]
    n981 = Select(t=i8 18, s=w1113, f=w1112) -> (s? t:f=w1117:i8)
    n982 = global write "Robot Global Data.vi" "Robot Lights"(w1117) -> ()
    n983 = Wait (ms)(milliseconds to wait=u32 100) -> ()  [unwired: 1 out]
  }
  n984 = while {
    stop <- FALSE stop-if-true
    # "Vision Processing\nTarget Distance Calculator"
    n985 = global read "Robot Global Data.vi" "Lime In View"() -> (w1120:bool)
    n986 = case shown="True" w1120 {
      frame False {
      }
      frame True {
        # "Manual Calibration"
        # "Mount height"
        # "Target height"
        # "Degrees to Radians\nConversion Factor"
        # "Mounting Angle"
        n987 = global read "Robot Global Data.vi" "Lime Y Angle"() -> (w1133:dbl)
        n988 = Divide(x=3.141592653589793, y=180.0) -> (x/y=w1135:dbl)
        n989 = Multiply(x=30.0, y=w1135) -> (x*y=w1131:dbl)
        n990 = Multiply(x=w1133, y=w1135) -> (x*y=w1132:dbl)
        n991 = Subtract(x=104.0, y=9.5) -> (x-y=w1126:dbl)
        n992 = Add(x=w1131, y=w1132) -> (x+y=w1130:dbl)
        n993 = Tangent(1:w1130) -> (0:w1127:dbl)
        n994 = global read "Robot Global Data.vi" "V02"() -> (w1121:dbl)
        n995 = Add(x=-40.0 ("y"), y=w1121) -> (x+y=w1122:dbl)
        n996 = Divide(x=w1126, y=w1127) -> (x/y=w1125:dbl)
        n997 = Add(x=w1125, y=w1122) -> (x+y=w1124:dbl)
        n998 = global write "Robot Global Data.vi" "Target Dist"(w1124) -> ()
      }
    }
    n999 = Wait (ms)(milliseconds to wait=u32 100) -> ()  [unwired: 1 out]
  }
  n1000 = while {
    stop <- FALSE stop-if-true
    # "Write to Dashboard"
    n1001 = global read "Robot Global Data.vi" "Tee Lo Power"() -> (w1154:bool)
    n1002 = global read "Robot Global Data.vi" "Locked On"() -> (w1159:bool)
    n1003 = global read "Robot Global Data.vi" "OC_Shoot"() -> (w1150:bool)
    n1004 = global read "Robot Global Data.vi" "DC_Shoot"() -> (w1149:bool)
    n1005 = global read "Robot Global Data.vi" "Centering"() -> (w1158:bool)
    n1006 = global read "Robot Global Data.vi" "Climb On"() -> (w1151:bool)
    n1007 = global read "Robot Global Data.vi" "Precision"() -> (w1162:bool)
    n1008 = global read "Robot Global Data.vi" "VX Align"() -> (w1155:bool)
    n1009 = global read "Robot Global Data.vi" "VY Align"() -> (w1156:bool)
    n1010 = global read "Robot Global Data.vi" "Tracking"() -> (w1157:bool)
    n1011 = global read "Robot Global Data.vi" "Tee-Out"() -> (w1153:bool)
    n1012 = global read "Robot Global Data.vi" "Rumble"() -> (w1160:bool)
    n1013 = global read "Robot Global Data.vi" "Reverse"() -> (w1161:bool)
    n1014 = global read "Robot Global Data.vi" "TB_Out"() -> (w1152:bool)
    n1015 = Insert Into Array(array=bool[] [], new element #1=w1162, new element #2=w1161, new element #3=w1160, new element #4=w1149, new element #5=w1150, new element #6=w1151, new element #7=w1152, new element #8=w1153, new element #9=w1154, new element #10=w1155, new element #11=w1156, new element #12=w1157, new element #13=w1158, new element #14=w1159) -> (w1167:bool[])  [unwired: 1 in]
    n1016 = call-poly <vilib>:"NT Write Value.vi"("Boolean Array"=w1167, "Name"="D_R Boolean Array") -> ()  [unwired: 9 in, 1 out]
    n1017 = global read "Robot Global Data.vi" "Desired Tee_Pot"() -> (w1163:dbl)
    n1018 = global read "Robot Global Data.vi" "Flywheel Speed"() -> (w1140:dbl)
    n1019 = global read "Robot Global Data.vi" "Desired Speed"() -> (w1139:dbl)
    n1020 = global read "Robot Global Data.vi" "Robot Lights"() -> (w1148:i8)
    n1021 = global read "Robot Global Data.vi" "Carriage Pos"() -> (w1144:T1)
    n1022 = global read "Robot Global Data.vi" "Drv Dist Av"() -> (w1174:dbl)
    n1023 = global read "Robot Global Data.vi" "Drv Spd Av"() -> (w1171:dbl)
    n1024 = global read "Robot Global Data.vi" "Target Dist"() -> (w1147:dbl)
    n1025 = global read "Robot Global Data.vi" "Intake Pwr"() -> (w1141:dbl)
    n1026 = global read "Robot Global Data.vi" "Drv Dist R"() -> (w1173:dbl)
    n1027 = global read "Robot Global Data.vi" "Drv Spd R"() -> (w1170:dbl)
    n1028 = global read "Robot Global Data.vi" "Drv Dist L"() -> (w1175:dbl)
    n1029 = global read "Robot Global Data.vi" "Drv Spd L"() -> (w1172:dbl)
    n1030 = global read "Robot Global Data.vi" "Auto TS"() -> (w1164:i8)
    n1031 = global read "Robot Global Data.vi" "Tee_Pot"() -> (w1138:dbl)
    n1032 = global read "Robot Global Data.vi" "Lime X"() -> (w1145:dbl)
    n1033 = global read "Robot Global Data.vi" "Lime Y"() -> (w1146:dbl)
    n1034 = global read "Robot Global Data.vi" "TBar R"() -> (w1143:dbl)
    n1035 = global read "Robot Global Data.vi" "TBar L"() -> (w1142:dbl)
    n1036 = Insert Into Array(array=dbl[] [], new element #1=w1175, new element #2=w1174, new element #3=w1173, new element #4=w1172, new element #5=w1171, new element #6=w1170, new element #7=w1164, new element #8=w1163, new element #9=w1138, new element #10=w1139, new element #11=w1140, new element #12=w1141, new element #13=w1142, new element #14=w1143, new element #15=w1144, new element #16=w1145, new element #17=w1146, new element #18=w1147, new element #19=w1148) -> (w1176:dbl[])  [unwired: 1 in]
    n1037 = call-poly <vilib>:"NT Write Value.vi"("Numeric Array"=w1176, "Name"="D_R Numeric Array") -> ()  [unwired: 9 in, 1 out]
    n1038 = global read "Robot Global Data.vi" "Drive"() -> (w1177:string)
    n1039 = Insert Into Array(array=string[] [], new element=w1177) -> (w1180:string[])  [unwired: 1 in]
    n1040 = call-poly <vilib>:"NT Write Value.vi"("String Array"=w1180, "Name"="D_R String Array") -> ()  [unwired: 9 in, 1 out]
    n1041 = Wait (ms)(milliseconds to wait=u32 50) -> ()  [unwired: 1 out]
  }
  n1042 = while {
    stop <- FALSE stop-if-true
    # "Diagnostic Robot Main LEDs"
    n1043 = global read "Robot Global Data.vi" "LED Reset"() -> (w1185:bool)
    n1044 = case shown="True" w1185 {
      frame False {
      }
      frame True {
        n1045 = flat-sequence {
          frame #0 {
            w1186 = FALSE
            n1046 = global write "Robot Global Data.vi" "LED 1"(w1186) -> ()
            n1047 = global write "Robot Global Data.vi" "LED 2"(w1186) -> ()
            n1048 = global write "Robot Global Data.vi" "LED 3"(w1186) -> ()
            n1049 = global write "Robot Global Data.vi" "LED 4"(w1186) -> ()
            n1050 = global write "Robot Global Data.vi" "LED 5"(w1186) -> ()
            n1051 = global write "Robot Global Data.vi" "LED 6"(w1186) -> ()
            n1052 = global write "Robot Global Data.vi" "LED 7"(w1186) -> ()
            n1053 = global write "Robot Global Data.vi" "LED 8"(w1186) -> ()
            n1054 = global write "Robot Global Data.vi" "LED 9"(w1186) -> ()
          }
          frame #1 {
            n1055 = global write "Robot Global Data.vi" "LED Reset"(FALSE ("LED Reset")) -> ()
          }
        }
      }
    }
    n1056 = Wait (ms)(milliseconds to wait=u32 100) -> ()  [unwired: 1 out]
  }
  n1057 = disable-structure shown="Disabled" {
    frame Disabled {
      n1058 = global read "Robot Global Data.vi" "TBar L"() -> (w1193:dbl)
      n1059 = global read "Robot Global Data.vi" "TBar R"() -> (w1192:dbl)
      n1060 = global read "Robot Global Data.vi" "TBar L"() -> (w1196:dbl)
      n1061 = Subtract(x=w1193, y=w1192) -> (x-y=w1191:dbl)
      n1062 = Absolute Value(x=w1191) -> (abs(x)=w1190:dbl)
      n1063 = Greater?(x=w1196, y=90.0) -> (0:w1188:bool)
      n1064 = Greater?(x=w1190, y=5.0) -> (0:w1189:bool)
      n1065 = And(x=w1188, y=w1189) -> ()  [unwired: 1 out]
    }
    frame Enabled {
    }
  }
  n1066 = call <vilib>:"CTRE_Phoenix_MotorControl_RefNumRegistryGet.vi"("refnum name"="B_Drv R1") -> ("PhoenixMotorControlDevRef"=w12:T15)  [unwired: 9 in, 1 out]
  n1067 = call <vilib>:"CTRE_Phoenix_MotorControl_RefNumRegistryGet.vi"("refnum name"="B_Drv R2") -> ("PhoenixMotorControlDevRef"=w13:T15)  [unwired: 9 in, 1 out]
  n1068 = call <vilib>:"CTRE_Phoenix_MotorControl_RefNumRegistryGet.vi"("refnum name"="B_Drv L1") -> ("PhoenixMotorControlDevRef"=w14:T15)  [unwired: 9 in, 1 out]
  n1069 = call <vilib>:"CTRE_Phoenix_MotorControl_RefNumRegistryGet.vi"("refnum name"="B_Drv L2") -> ("PhoenixMotorControlDevRef"=w11:T15)  [unwired: 9 in, 1 out]
  n1070 = while {
    stop <- FALSE stop-if-true
    w1213 = 10.0 ("y")
    w1214 = 1.2 ("y")
    w1215 = -1.2 ("y")
    w1216 = -10.0 ("y")
    w1212 = -100.0 ("y")
    w1211 = 100.0 ("y")
    # "Tee/Carriage Feedback Loop"
    n1071 = global read "Robot Global Data.vi" "Desired Tee_Pot"() -> (w1200:dbl)
    n1072 = global read "Robot Global Data.vi" "Tee_Pot"() -> (w1199:dbl)
    n1073 = Subtract(x=w1200, y=w1199) -> (x-y=w1201:dbl)
    n1074 = In Range and Coerce(upper limit=500.0, x=w1201, lower limit=w1211) -> (In Range?=w1204:bool)  [unwired: 1 out]
    n1075 = In Range and Coerce(upper limit=w1211, x=w1201, lower limit=w1213) -> (In Range?=w1205:bool)  [unwired: 1 out]
    n1076 = In Range and Coerce(upper limit=w1213, x=w1201, lower limit=w1214) -> (In Range?=w1206:bool)  [unwired: 1 out]
    n1077 = In Range and Coerce(upper limit=w1214, x=w1201, lower limit=w1215) -> (In Range?=w1207:bool)  [unwired: 1 out]
    n1078 = In Range and Coerce(upper limit=w1215, x=w1201, lower limit=w1216) -> (In Range?=w1208:bool)  [unwired: 1 out]
    n1079 = In Range and Coerce(upper limit=w1216, x=w1201, lower limit=w1212) -> (In Range?=w1209:bool)  [unwired: 1 out]
    n1080 = In Range and Coerce(upper limit=w1212, x=w1201, lower limit=-500.0) -> (In Range?=w1210:bool)  [unwired: 1 out]
    n1081 = case shown="True" w1204 {
      frame False {
      }
      frame True {
        n1082 = global write "Robot Global Data.vi" "Auto Tee Pwr"(0.75 ("Tee_Pot")) -> ()
      }
    }
    n1083 = case shown="True" w1205 {
      frame False {
      }
      frame True {
        n1084 = global write "Robot Global Data.vi" "Auto Tee Pwr"(0.55 ("Tee_Pot")) -> ()
      }
    }
    n1085 = case shown="True" w1206 {
      frame False {
      }
      frame True {
        n1086 = global write "Robot Global Data.vi" "Auto Tee Pwr"(0.15 ("Tee_Pot")) -> ()
      }
    }
    n1087 = case shown="True" w1207 {
      frame False {
      }
      frame True {
        n1088 = global write "Robot Global Data.vi" "Auto Tee Pwr"(0.0 ("Tee_Pot")) -> ()
      }
    }
    n1089 = case shown="True" w1208 {
      frame False {
      }
      frame True {
        n1090 = global write "Robot Global Data.vi" "Auto Tee Pwr"(-0.15 ("Tee_Pot")) -> ()
      }
    }
    n1091 = case shown="True" w1209 {
      frame False {
      }
      frame True {
        n1092 = global write "Robot Global Data.vi" "Auto Tee Pwr"(-0.55 ("Tee_Pot")) -> ()
      }
    }
    n1093 = case shown="True" w1210 {
      frame False {
      }
      frame True {
        n1094 = global write "Robot Global Data.vi" "Auto Tee Pwr"(-0.75 ("Tee_Pot")) -> ()
      }
    }
    n1095 = Wait (ms)(milliseconds to wait=u32 50) -> ()  [unwired: 1 out]
  }
  n1096 = while {
    stop <- FALSE stop-if-true
    # "Flywheel Feedback Loop"
    n1097 = global read "Robot Global Data.vi" "Fly_Adjust"() -> (w1225:bool)
    n1098 = global read "Robot Global Data.vi" "Flywheel On"() -> (w1228:bool)
    n1099 = call <vilib>:"WPI_DriverStationOutputsEnabled.vi"() -> ("OutputsEnabled?"=w1227:bool)  [unwired: 10 in, 1 out]
    n1100 = Not(x=w1225) -> (.not. x?=w1224:bool)
    n1101 = Compound Arithmetic op=AND(w1224, w1228, w1227) -> (w1226:bool)
    n1102 = case shown="True" w1226 {
      frame False {
        n1103 = global read "Robot Global Data.vi" "Fly_Adjust"() -> (w1232:bool)
        n1104 = Not(x=w1232) -> (.not. x?=w1231:bool)
        n1105 = case shown="True" w1231 {
          frame False {
          }
          frame True {
            n1106 = global write "Robot Global Data.vi" "Flywheel Power"(0.0 ("Flywheel Power")) -> ()
          }
        }
      }
      frame True {
        n1107 = global read "Robot Global Data.vi" "OC_Shoot Off"() -> (w1234:bool)
        n1108 = Not(x=w1234) -> (.not. x?=w1235:bool)
        n1109 = case shown="True" w1235 {
          frame False {
            n1110 = global read "Robot Global Data.vi" "Flywheel Power"() -> (w1236:dbl)
            n1111 = global write "Robot Global Data.vi" "Flywheel Power"(w1236) -> ()
          }
          frame True {
            w1238 = -6000.0 ("lower limit")
            w1241 = 6000.0 ("lower limit")
            w1246 = -4000.0 ("lower limit")
            w1247 = -3000.0 ("lower limit")
            w1248 = -500.0 ("lower limit")
            w1249 = 4000.0 ("lower limit")
            w1250 = 3000.0 ("lower limit")
            w1251 = 500.0 ("lower limit")
            n1112 = global read "Robot Global Data.vi" "Flywheel Speed"() -> (w1244:dbl)
            n1113 = global read "Robot Global Data.vi" "Desired Speed"() -> (w1245:dbl)
            n1114 = Subtract(x=w1245, y=w1244) -> (x-y=w1239:dbl)
            n1115 = In Range and Coerce(upper limit=w1249, x=w1239, lower limit=w1250) -> (In Range?=w1257:bool)  [unwired: 1 out]
            n1116 = In Range and Coerce(upper limit=w1247, x=w1239, lower limit=w1246) -> (In Range?=w1253:bool)  [unwired: 1 out]
            n1117 = In Range and Coerce(upper limit=w1246, x=w1239, lower limit=w1238) -> (In Range?=w1252:bool)  [unwired: 1 out]
            n1118 = In Range and Coerce(upper limit=w1238, x=w1239, lower limit=-100000.0) -> (In Range?=w1243:bool)  [unwired: 1 out]
            n1119 = In Range and Coerce(upper limit=100000.0, x=w1239, lower limit=w1241) -> (In Range?=w1242:bool)  [unwired: 1 out]
            n1120 = In Range and Coerce(upper limit=w1241, x=w1239, lower limit=w1249) -> (In Range?=w1258:bool)  [unwired: 1 out]
            n1121 = In Range and Coerce(upper limit=w1250, x=w1239, lower limit=w1251) -> (In Range?=w1256:bool)  [unwired: 1 out]
            n1122 = In Range and Coerce(upper limit=w1251, x=w1239, lower limit=w1248) -> (In Range?=w1255:bool)  [unwired: 1 out]
            n1123 = In Range and Coerce(upper limit=w1248, x=w1239, lower limit=w1247) -> (In Range?=w1254:bool)  [unwired: 1 out]
            n1124 = case shown="True" w1258 {
              frame False {
              }
              frame True {
                n1125 = global read "Robot Global Data.vi" "Flywheel Power"() -> (w1282:dbl)
                n1126 = Add(x=0.05 ("Turret Swiv Speed"), y=w1282) -> (x+y=w1280:dbl)
                n1127 = global write "Robot Global Data.vi" "Flywheel Power"(w1280) -> ()
              }
            }
            n1128 = case shown="True" w1257 {
              frame False {
              }
              frame True {
                n1129 = global read "Robot Global Data.vi" "Flywheel Power"() -> (w1279:dbl)
                n1130 = Add(x=0.02 ("Turret Swiv Speed"), y=w1279) -> (x+y=w1277:dbl)
                n1131 = global write "Robot Global Data.vi" "Flywheel Power"(w1277) -> ()
              }
            }
            n1132 = case shown="True" w1256 {
              frame False {
              }
              frame True {
                n1133 = global read "Robot Global Data.vi" "Flywheel Power"() -> (w1276:dbl)
                n1134 = Add(x=0.0125 ("Turret Swiv Speed"), y=w1276) -> (x+y=w1274:dbl)
                n1135 = global write "Robot Global Data.vi" "Flywheel Power"(w1274) -> ()
              }
            }
            n1136 = case shown="True" w1255 {
              frame False {
              }
              frame True {
                n1137 = global read "Robot Global Data.vi" "Flywheel Power"() -> (w1273:dbl)
                n1138 = Add(x=0.0 ("Turret Swiv Speed"), y=w1273) -> (x+y=w1271:dbl)
                n1139 = global write "Robot Global Data.vi" "Flywheel Power"(w1271) -> ()
              }
            }
            n1140 = case shown="True" w1254 {
              frame False {
              }
              frame True {
                n1141 = global read "Robot Global Data.vi" "Flywheel Power"() -> (w1270:dbl)
                n1142 = Add(x=-0.0125 ("Turret Swiv Speed"), y=w1270) -> (x+y=w1268:dbl)
                n1143 = global write "Robot Global Data.vi" "Flywheel Power"(w1268) -> ()
              }
            }
            n1144 = case shown="True" w1253 {
              frame False {
              }
              frame True {
                n1145 = global read "Robot Global Data.vi" "Flywheel Power"() -> (w1267:dbl)
                n1146 = Add(x=-0.02 ("Turret Swiv Speed"), y=w1267) -> (x+y=w1265:dbl)
                n1147 = global write "Robot Global Data.vi" "Flywheel Power"(w1265) -> ()
              }
            }
            n1148 = case shown="True" w1252 {
              frame False {
              }
              frame True {
                n1149 = global read "Robot Global Data.vi" "Flywheel Power"() -> (w1264:dbl)
                n1150 = Add(x=-0.05 ("Turret Swiv Speed"), y=w1264) -> (x+y=w1262:dbl)
                n1151 = global write "Robot Global Data.vi" "Flywheel Power"(w1262) -> ()
              }
            }
            n1152 = case shown="True" w1243 {
              frame False {
              }
              frame True {
                n1153 = global read "Robot Global Data.vi" "Flywheel Power"() -> (w1285:dbl)
                n1154 = Add(x=-0.1 ("Turret Swiv Speed"), y=w1285) -> (x+y=w1283:dbl)
                n1155 = global write "Robot Global Data.vi" "Flywheel Power"(w1283) -> ()
              }
            }
            n1156 = case shown="True" w1242 {
              frame False {
              }
              frame True {
                n1157 = global read "Robot Global Data.vi" "Flywheel Power"() -> (w1261:dbl)
                n1158 = Add(x=0.1 ("Turret Swiv Speed"), y=w1261) -> (x+y=w1259:dbl)
                n1159 = global write "Robot Global Data.vi" "Flywheel Power"(w1259) -> ()
              }
            }
          }
        }
      }
    }
    n1160 = Wait (ms)(milliseconds to wait=u32 200) -> ()  [unwired: 1 out]
  }
  n1161 = while {
    tunnel: w11 -> [w1336]
    tunnel: w12 -> [w1325]
    tunnel: w13 -> [w1335]
    tunnel: [w1334] -> _
    tunnel: [w1333] -> _
    tunnel: [w1332] -> _
    tunnel: [w1331] -> _
    tunnel: w14 -> [w1326]
    stop <- FALSE stop-if-true
    w1287 = T19 0 items=["PercentOutput"=0, "Position"=1, "Velocity"=2, "Current"=3, "Follower"=5, "MotionProfile"=6, "MotionMagic"=7, "MotionProfileArc"=10, "Disabled"=15] ("Control Mode")
    w1323 = 14575.0
    w1324 = 1457.5
    # "Ratios for 4\" Wheels\n3900\n390"
    # "Ratios for 4\" Wheels"
    # "in Ft per Sec"
    # "Gearbox\nDirection\nCalibration"
    # "Drive System"
    # "in Ft"
    # "Default averages 64 samples over 100ms"
    # "Ratios for 6\" Wheels\n2600\n260"
    n1162 = global read "Robot Global Data.vi" "Drive"() -> (w1304:string)
    n1163 = global read "Robot Global Data.vi" "D_Enc-R"() -> (w1293:bool)
    n1164 = case shown="\"Cheesy\", Default" w1304 {
      tunnel: [w1372 w1389 w1404] -> w1314
      tunnel: [w1371 w1390 w1405] -> w1313
      frame "Cheesy", Default {
        w1362 = 1.0 ("upper limit")
        w1373 = -1.0 ("lower limit")
        w1374 = -1.0 ("lower limit")
        w1375 = 1.0 ("upper limit")
        # "1 = Steering\n2 = Gas/Brake"
        # "Cheesy"
        n1165 = disable-structure shown="Disabled" {
          frame Disabled {
            n1166 = global read "Robot Global Data.vi" "Turn Cal"() -> ()  [unwired: 1 out]
          }
          frame Enabled {
          }
        }
        n1167 = global read "Robot Global Data.vi" "Drv Input 1"() -> (w1354:dbl)
        n1168 = global read "Robot Global Data.vi" "Drv Input 2"() -> (w1355:dbl)
        n1169 = global read "Robot Global Data.vi" "Drift Cal"() -> (w1356:dbl)
        n1170 = Negate(x=w1355) -> (-x=w1357:dbl)
        n1171 = Absolute Value(x=w1354) -> (abs(x)=w1365:dbl)
        n1172 = Absolute Value(x=w1357) -> (abs(x)=w1370:dbl)
        n1173 = Greater Or Equal?(x=w1365, y=w1356) -> (x >= y?=w1366:bool)
        n1174 = Greater Or Equal?(x=w1370, y=w1356) -> (x >= y?=w1369:bool)
        n1175 = Select(t=w1354, s=w1366, f=0.0) -> (s? t:f=w1363:dbl)
        n1176 = Select(t=w1357, s=w1369, f=0.0) -> (s? t:f=w1364:dbl)
        n1177 = In Range and Coerce(upper limit=w1375, x=w1363, lower limit=w1374) -> (coerced(x)=w1359:dbl)  [unwired: 1 out]
        n1178 = In Range and Coerce(upper limit=w1375, x=w1364, lower limit=w1374) -> (coerced(x)=w1360:dbl)  [unwired: 1 out]
        n1179 = Add(x=w1359, y=w1360) -> (x+y=w1361:dbl)
        n1180 = Subtract(x=w1359, y=w1360) -> (x-y=w1358:dbl)
        n1181 = In Range and Coerce(upper limit=w1362, x=w1361, lower limit=w1373) -> (coerced(x)=w1372:dbl)  [unwired: 1 out]
        n1182 = In Range and Coerce(upper limit=w1362, x=w1358, lower limit=w1373) -> (coerced(x)=w1371:dbl)  [unwired: 1 out]
      }
      frame "Arcade" {
        w1395 = 1.0 ("upper limit")
        w1396 = -1.0 ("lower limit")
        w1397 = -1.0 ("lower limit")
        w1398 = 1.0 ("upper limit")
        # "1 = Steering\n2 = Gas/Brake"
        # "Arcade"
        n1183 = global read "Robot Global Data.vi" "Drv Input 1"() -> (w1379:dbl)
        n1184 = global read "Robot Global Data.vi" "Drv Input 2"() -> (w1378:dbl)
        n1185 = global read "Robot Global Data.vi" "Drift Cal"() -> (w1376:dbl)
        n1186 = global read "Robot Global Data.vi" "Turn Cal"() -> (w1377:dbl)
        n1187 = Absolute Value(x=w1379) -> (abs(x)=w1383:dbl)
        n1188 = Absolute Value(x=w1378) -> (abs(x)=w1388:dbl)
        n1189 = Multiply(x=w1377, y=w1379) -> (x*y=w1382:dbl)
        n1190 = Greater Or Equal?(x=w1383, y=w1376) -> (x >= y?=w1384:bool)
        n1191 = Greater Or Equal?(x=w1388, y=w1376) -> (x >= y?=w1387:bool)
        n1192 = Select(t=w1382, s=w1384, f=0.0) -> (s? t:f=w1380:dbl)
        n1193 = Select(t=w1378, s=w1387, f=0.0) -> (s? t:f=w1381:dbl)
        n1194 = In Range and Coerce(upper limit=w1398, x=w1380, lower limit=w1397) -> (coerced(x)=w1392:dbl)  [unwired: 1 out]
        n1195 = In Range and Coerce(upper limit=w1398, x=w1381, lower limit=w1397) -> (coerced(x)=w1393:dbl)  [unwired: 1 out]
        n1196 = Add(x=w1392, y=w1393) -> (x+y=w1394:dbl)
        n1197 = Subtract(x=w1392, y=w1393) -> (x-y=w1391:dbl)
        n1198 = In Range and Coerce(upper limit=w1395, x=w1394, lower limit=w1396) -> (coerced(x)=w1389:dbl)  [unwired: 1 out]
        n1199 = In Range and Coerce(upper limit=w1395, x=w1391, lower limit=w1396) -> (coerced(x)=w1390:dbl)  [unwired: 1 out]
      }
      frame "Tank" {
        w1406 = 1.0 ("upper limit")
        w1407 = -1.0 ("lower limit")
        # "Tank"
        n1200 = global read "Robot Global Data.vi" "Drv Input 1"() -> (w1400:dbl)
        n1201 = global read "Robot Global Data.vi" "Drv Input 2"() -> (w1399:dbl)
        n1202 = global read "Robot Global Data.vi" "Drift Cal"() -> (w1401:dbl)
        n1203 = Absolute Value(x=w1400) -> (abs(x)=w1413:dbl)
        n1204 = Absolute Value(x=w1399) -> (abs(x)=w1410:dbl)
        n1205 = Greater Or Equal?(x=w1413, y=w1401) -> (x >= y?=w1412:bool)
        n1206 = Greater Or Equal?(x=w1410, y=w1401) -> (x >= y?=w1411:bool)
        n1207 = Select(t=w1400, s=w1412, f=0.0) -> (s? t:f=w1414:dbl)
        n1208 = Select(t=w1399, s=w1411, f=0.0) -> (s? t:f=w1402:dbl)
        n1209 = Negate(x=w1414) -> (-x=w1403:dbl)
        n1210 = In Range and Coerce(upper limit=w1406, x=w1403, lower limit=w1407) -> (coerced(x)=w1404:dbl)  [unwired: 1 out]
        n1211 = In Range and Coerce(upper limit=w1406, x=w1402, lower limit=w1407) -> (coerced(x)=w1405:dbl)  [unwired: 1 out]
      }
    }
    n1212 = case shown="True" w1293 {
      tunnel: w1326 -> [w1416 w1422]
      tunnel: [w1416 w1421] -> w1320
      tunnel: w1325 -> [w1415 w1419]
      tunnel: [w1415 w1418] -> w1321
      frame False {
      }
      frame True {
        n1213 = global write "Robot Global Data.vi" "D_Enc-R"(FALSE ("D_Enc-R TS")) -> ()
        n1214 = call-poly <vilib>:"CTRE_Phoenix_MotorControl_SetIntegratedSensorPosition_TalonFX_Polymorphic.vi"("New Position"=0.0, "PhoenixMotorControlDevRef"=w1419) -> ("PhoenixMotorControlDevRef"=w1418:T15)  [unwired: 8 in, 1 out]
        n1215 = call-poly <vilib>:"CTRE_Phoenix_MotorControl_SetIntegratedSensorPosition_TalonFX_Polymorphic.vi"("New Position"=0.0, "PhoenixMotorControlDevRef"=w1422) -> ("PhoenixMotorControlDevRef"=w1421:T15)  [unwired: 8 in, 1 out]
      }
    }
    n1216 = call-poly <vilib>:"CTRE_Phoenix_MotorController_Get_TalonFX.vi"("PhoenixMotorControlDevRef"=w1320) -> ("PhoenixMotorControlDevRef"=w1330:T15, "Position"=w1319:dbl, "Velocity"=w1288:dbl)  [unwired: 10 in, 2 out]
    n1217 = call-poly <vilib>:"CTRE_Phoenix_MotorController_Get_TalonFX.vi"("PhoenixMotorControlDevRef"=w1321) -> ("PhoenixMotorControlDevRef"=w1306:T15, "Position"=w1316:dbl, "Velocity"=w1289:dbl)  [unwired: 10 in, 2 out]
    n1218 = global read "Robot Global Data.vi" "A Drv"() -> (w1292:bool)
    n1219 = global read "Robot Global Data.vi" "Reverse"() -> (w1303:bool)
    n1220 = global read "Robot Global Data.vi" "Precision"() -> (w1302:bool)
    n1221 = Negate(x=w1319) -> (-x=w1317:dbl)
    n1222 = Negate(x=w1289) -> (-x=w1318:dbl)
    n1223 = case shown="True" w1302 {
      tunnel: w1314 -> [w1343 w1349]
      tunnel: [w1343 w1348] -> w1312
      tunnel: w1313 -> [w1342 w1347]
      tunnel: [w1342 w1346] -> w1311
      frame False {
      }
      frame True {
        # "Precision\nDrive"
        n1224 = Multiply(x=w1349, y=0.5 ("upper limit")) -> (x*y=w1348:dbl)
        n1225 = Multiply(x=w1347, y=0.5) -> (x*y=w1346:dbl)
      }
    }
    n1226 = Divide(x=w1317, y=w1323) -> (x/y=w1295:dbl)
    n1227 = Divide(x=w1316, y=w1323) -> (x/y=w1294:dbl)
    n1228 = Divide(x=w1288, y=w1324) -> (x/y=w1297:dbl)
    n1229 = Divide(x=w1318, y=w1324) -> (x/y=w1296:dbl)
    n1230 = global read "Robot Global Data.vi" "Drv-L-Out"() -> (w1291:dbl)
    n1231 = global read "Robot Global Data.vi" "Drv-R-Out"() -> (w1290:dbl)
    n1232 = Add(x=w1295, y=w1294) -> (x+y=w1329:dbl)
    n1233 = Add(x=w1297, y=w1296) -> (x+y=w1327:dbl)
    n1234 = case shown="True" w1303 {
      tunnel: [w1339 w1341] -> w1310
      tunnel: [w1338 w1340] -> w1309
      tunnel: w1312 -> [w1339 w1340]
      tunnel: w1311 -> [w1338 w1341]
      frame False {
      }
      frame True {
        # "Rev"
      }
    }
    n1235 = Divide(x=w1329, y=2.0) -> (x/y=w1299:dbl)
    n1236 = Divide(x=w1327, y=2.0) -> (x/y=w1298:dbl)
    n1237 = case shown="True" w1292 {
      tunnel: [w1351 w1353] -> w1308
      tunnel: [w1350 w1352] -> w1307
      tunnel: w1310 -> [w1351 _]
      tunnel: w1309 -> [w1350 _]
      frame False {
        # "Normal\nController\nDriving"
      }
      frame True {
        # "Autonomous\nDriving"
        n1238 = global read "Robot Global Data.vi" "A Drv-L"() -> (w1353:dbl)
        n1239 = global read "Robot Global Data.vi" "A Drv-R"() -> (w1352:dbl)
      }
    }
    n1240 = global write "Robot Global Data.vi" "Drv Dist L"(w1295) -> ()
    n1241 = global write "Robot Global Data.vi" "Drv Dist Av"(w1299) -> ()
    n1242 = global write "Robot Global Data.vi" "Drv Dist R"(w1294) -> ()
    n1243 = global write "Robot Global Data.vi" "Drv Spd L"(w1297) -> ()
    n1244 = global write "Robot Global Data.vi" "Drv Spd Av"(w1298) -> ()
    n1245 = global write "Robot Global Data.vi" "Drv Spd R"(w1296) -> ()
    n1246 = Multiply(x=w1308, y=1.0) -> (x*y=w1301:dbl)
    n1247 = Multiply(x=w1307, y=1.0) -> (x*y=w1300:dbl)
    n1248 = global write "Robot Global Data.vi" "Drv-L-Out"(w1301) -> ()
    n1249 = global write "Robot Global Data.vi" "Drv-R-Out"(w1300) -> ()
    n1250 = call <vilib>:"CTRE_Phoenix_MotorControl_Set.vi"("Output"=w1291, "Control Mode"=w1287, "PhoenixMotorControlDevRef"=w1330) -> ("PhoenixMotorControlDevRef"=w1331:T15)  [unwired: 7 in, 1 out]
    n1251 = call <vilib>:"CTRE_Phoenix_MotorControl_Set.vi"("Output"=w1291, "Control Mode"=w1287, "PhoenixMotorControlDevRef"=w1336) -> ("PhoenixMotorControlDevRef"=w1332:T15)  [unwired: 7 in, 1 out]
    n1252 = call <vilib>:"CTRE_Phoenix_MotorControl_Set.vi"("Output"=w1290, "Control Mode"=w1287, "PhoenixMotorControlDevRef"=w1306) -> ("PhoenixMotorControlDevRef"=w1333:T15)  [unwired: 7 in, 1 out]
    n1253 = call <vilib>:"CTRE_Phoenix_MotorControl_Set.vi"("Output"=w1290, "Control Mode"=w1287, "PhoenixMotorControlDevRef"=w1335) -> ("PhoenixMotorControlDevRef"=w1334:T15)  [unwired: 7 in, 1 out]
    n1254 = Wait (ms)(milliseconds to wait=u32 20) -> ()  [unwired: 1 out]
  }
  n1255 = disable-structure shown="Disabled" {
    frame Disabled {
      n1256 = case shown="True" FALSE {
        tunnel: _ -> [w1426 w1438]
        tunnel: _ -> [w1425 w1428]
        tunnel: [w1426 w1437] -> _
        tunnel: [w1425 w1427] -> _
        frame False {
        }
        frame True {
          n1257 = global read "Robot Global Data.vi" "TBar L"() -> (w1432:dbl)
          n1258 = global read "Robot Global Data.vi" "TBar L"() -> (w1435:dbl)
          n1259 = global read "Robot Global Data.vi" "TBar R"() -> (w1434:dbl)
          n1260 = global read "Robot Global Data.vi" "TBar R"() -> (w1433:dbl)
          n1261 = Greater?(x=w1432, y=w1433) -> (0:w1431:bool)
          n1262 = Less?(x=w1435, y=w1434) -> (x < y?=w1436:bool)
          n1263 = Select(t=0.0, s=w1436, f=w1438) -> (s? t:f=w1437:dbl)
          n1264 = Select(t=0.0, s=w1431, f=w1428) -> (s? t:f=w1427:dbl)
        }
      }
    }
    frame Enabled {
    }
  }
  n1265 = disable-structure shown="Disabled" {
    frame Disabled {
      n1266 = call <vilib>:"WPI_SolenoidRefNum Registry Get.vi"("refnum name"="B_Shifter") -> ("SolenoidDevRef"=w1439:T9)  [unwired: 9 in, 1 out]
      n1267 = while {
        tunnel: w1439 -> [w1443]
        tunnel: [w1442] -> _
        stop <- FALSE stop-if-true
        # "Gear Box Shifters (0, 1)"
        n1268 = global read "Robot Global Data.vi" "Precision"() -> (w1444:bool)
        n1269 = case shown="True" w1444 {
          tunnel: [WPI_SolenoidValue."Forward" ("Value") WPI_SolenoidValue."Reverse" ("Value")] -> w1446
          frame False {
          }
          frame True {
          }
        }
        n1270 = global read "Robot Global Data.vi" "High Gear"() -> (w1447)
        n1271 = Select(t=w1446, s=w1447, f=WPI_SolenoidValue."Reverse" ("Value")) -> (s? t:f=w1441:T11)
        n1272 = call-poly <vilib>:"WPI_SolenoidSet.vi"("Value"=w1441, "SolenoidDevRef"=w1443) -> ("SolenoidDevRef"=w1442:T9)  [unwired: 8 in, 1 out]
        n1273 = Wait (ms)(milliseconds to wait=u32 100) -> ()  [unwired: 1 out]
      }
    }
    frame Enabled {
    }
  }
  n1274 = disable-structure shown="Disabled" {
    frame Disabled {
      n1275 = call <vilib>:"WPI_RelayRefNum Registry Get.vi"("refnum name"="B_Halo On") -> ("RelayDevRef"=w1452:T24)  [unwired: 9 in, 1 out]
      n1276 = while {
        tunnel: w1452 -> [w1455]
        tunnel: [w1454] -> _
        stop <- FALSE stop-if-true
        # "Halo On/Off (Relay 0)\nNote:  Blinks.  Use DIO Instead"
        n1277 = global read "Robot Global Data.vi" "Halo On"() -> (w1459:bool)
        n1278 = Select(t=WPI_SolenoidValue."Forward" ("Value"), s=w1459, f=WPI_SolenoidValue."Off" ("Value")) -> (s? t:f=w1456:T11)
        n1279 = call <vilib>:"WPI_RelaySet.vi"("RelayValue"=w1456, "RelayDevRef"=w1455) -> ("RelayDevRef"=w1454:T24)  [unwired: 8 in, 1 out]
        n1280 = Wait (ms)(milliseconds to wait=u32 100) -> ()  [unwired: 1 out]
      }
    }
    frame Enabled {
    }
  }
  n1281 = disable-structure shown="Disabled" {
    frame Disabled {
      # "Speed Adjusted Turn Calibration"
      n1282 = global read "Robot Global Data.vi" "Drv Spd Av"() -> (w1463:dbl)
      n1283 = Absolute Value(x=w1463) -> (abs(x)=w1470:dbl)
      n1284 = Divide(x=w1470, y=25.0) -> (x/y=w1466:dbl)
      n1285 = In Range and Coerce(upper limit=0.8, x=w1466, lower limit=0.0) -> (coerced(x)=w1467:dbl)  [unwired: 1 out]
      n1286 = Subtract(x=1.0, y=w1467) -> (x-y=w1462:dbl)
      n1287 = global write "Robot Global Data.vi" "Turn Cal"(w1462) -> ()
    }
    frame Enabled {
    }
  }
  n1288 = while {
    stop <- FALSE stop-if-true
    # "Vision Processing Y-Axis\n[Auto Centering]\n! Untested"
    n1289 = global read "Robot Global Data.vi" "VY Align"() -> (w1472:bool)
    n1290 = global read "Robot Global Data.vi" "Climb On"() -> (w1474:bool)
    n1291 = Not(x=w1474) -> (.not. x?=w1471:bool)
    n1292 = Compound Arithmetic op=AND(w1472, w1471) -> (w1473:bool)
    n1293 = case shown="True" w1473 {
      frame False {
      }
      frame True {
        n1294 = flat-sequence {
          frame #0 {
            n1295 = global write "Robot Global Data.vi" "A Drv"(TRUE ("Rumble")) -> ()
            n1296 = global write "Robot Global Data.vi" "A Exit"(FALSE ("Rumble")) -> ()
            n1297 = global write "Robot Global Data.vi" "Centering"(TRUE ("Centering")) -> ()
          }
          frame #1 {
            w1480 = FALSE ("A Exit")
            n1298 = for {
              N: 100 -> [_]
              shift-right: [w1496] -> _
              shift-left: w1480 -> [w1495]
              shift-left: w1480 -> [w1494]
              shift-left: w1480 -> [w1493]
              shift-left: w1480 -> [w1492]
              stop <- w1505 stop-if-true
              w1498 = 0.2 ("y")
              w1506 = -4.0 ("y")
              w1507 = 4.0 ("y")
              w1513 = -10.0 ("y")
              w1485 = -24.0 ("lower limit")
              w1484 = 24.0 ("upper limit")
              w1514 = 10.0 ("y")
              # "To check if past four\niterations of loop has\nA Exit true; Aprrox.\nCentered"
              n1299 = global read "Robot Global Data.vi" "Desired Dist"() -> (w1489:dbl)
              n1300 = global read "Robot Global Data.vi" "Target Dist"() -> (w1490:dbl)
              n1301 = global read "Robot Global Data.vi" "Drv Input 1"() -> (w1501:dbl)
              n1302 = global read "Robot Global Data.vi" "Drv Input 2"() -> (w1503:dbl)
              n1303 = Wait (ms)(milliseconds to wait=u32 100) -> ()  [unwired: 1 out]
              n1304 = Compound Arithmetic op=AND(w1495, w1494, w1493, w1492) -> (w1491:bool)
              n1305 = Subtract(x=w1489, y=w1490) -> (x-y=w1486:dbl)
              n1306 = Absolute Value(x=w1501) -> (abs(x)=w1502:dbl)
              n1307 = Absolute Value(x=w1503) -> (abs(x)=w1504:dbl)
              n1308 = Greater?(x=w1502, y=w1498) -> (0:w1499:bool)
              n1309 = Greater?(x=w1504, y=w1498) -> (0:w1500:bool)
              n1310 = In Range and Coerce(upper limit=72.0, x=w1486, lower limit=w1484) -> (In Range?=w1487:bool)  [unwired: 1 out]
              n1311 = In Range and Coerce(upper limit=w1484, x=w1486, lower limit=w1514) -> (In Range?=w1510:bool)  [unwired: 1 out]
              n1312 = In Range and Coerce(upper limit=w1514, x=w1486, lower limit=w1507) -> (In Range?=w1511:bool)  [unwired: 1 out]
              n1313 = In Range and Coerce(upper limit=w1507, x=w1486, lower limit=w1506) -> (In Range?=w1512:bool)  [unwired: 1 out]
              n1314 = In Range and Coerce(upper limit=w1506, x=w1486, lower limit=w1513) -> (In Range?=w1509:bool)  [unwired: 1 out]
              n1315 = In Range and Coerce(upper limit=w1513, x=w1486, lower limit=w1485) -> (In Range?=w1508:bool)  [unwired: 1 out]
              n1316 = In Range and Coerce(upper limit=w1485, x=w1486, lower limit=-72.0) -> (In Range?=w1488:bool)  [unwired: 1 out]
              n1317 = Or(x=w1499, y=w1500) -> (x .or. y?=w1497:bool)
              n1318 = case shown="True" w1487 {
                frame False {
                }
                frame True {
                  w1516 = -0.3 ("A Drv-L")
                  n1319 = Negate(x=w1516) -> (-x=w1517:dbl)
                  n1320 = global write "Robot Global Data.vi" "A Drv-L"(w1516) -> ()
                  n1321 = global write "Robot Global Data.vi" "A Drv-R"(w1517) -> ()
                }
              }
              n1322 = case shown="True" w1509 {
                frame False {
                }
                frame True {
                  w1522 = 0.075 ("A Drv-L")
                  n1323 = Negate(x=w1522) -> (-x=w1523:dbl)
                  n1324 = global write "Robot Global Data.vi" "A Drv-L"(w1522) -> ()
                  n1325 = global write "Robot Global Data.vi" "A Drv-R"(w1523) -> ()
                }
              }
              n1326 = case shown="True" w1510 {
                frame False {
                }
                frame True {
                  w1528 = -0.15 ("A Drv-L")
                  n1327 = Negate(x=w1528) -> (-x=w1529:dbl)
                  n1328 = global write "Robot Global Data.vi" "A Drv-L"(w1528) -> ()
                  n1329 = global write "Robot Global Data.vi" "A Drv-R"(w1529) -> ()
                }
              }
              n1330 = case shown="True" w1511 {
                frame False {
                }
                frame True {
                  w1526 = -0.075 ("A Drv-L")
                  n1331 = Negate(x=w1526) -> (-x=w1527:dbl)
                  n1332 = global write "Robot Global Data.vi" "A Drv-L"(w1526) -> ()
                  n1333 = global write "Robot Global Data.vi" "A Drv-R"(w1527) -> ()
                }
              }
              n1334 = case shown="True" w1512 {
                frame False {
                }
                frame True {
                  w1524 = 0.0 ("4Bar Auto")
                  n1335 = global write "Robot Global Data.vi" "A Drv-L"(w1524) -> ()
                  n1336 = global write "Robot Global Data.vi" "A Drv-R"(w1524) -> ()
                  n1337 = global write "Robot Global Data.vi" "A Exit"(TRUE ("A Exit")) -> ()
                }
              }
              n1338 = case shown="True" w1508 {
                frame False {
                }
                frame True {
                  w1520 = 0.15 ("A Drv-L")
                  n1339 = Negate(x=w1520) -> (-x=w1521:dbl)
                  n1340 = global write "Robot Global Data.vi" "A Drv-L"(w1520) -> ()
                  n1341 = global write "Robot Global Data.vi" "A Drv-R"(w1521) -> ()
                }
              }
              n1342 = case shown="True" w1488 {
                frame False {
                }
                frame True {
                  w1518 = 0.3 ("A Drv-L")
                  n1343 = Negate(x=w1518) -> (-x=w1519:dbl)
                  n1344 = global write "Robot Global Data.vi" "A Drv-L"(w1518) -> ()
                  n1345 = global write "Robot Global Data.vi" "A Drv-R"(w1519) -> ()
                }
              }
              n1346 = Or(x=w1491, y=w1497) -> (x .or. y?=w1505:bool)
              n1347 = global read "Robot Global Data.vi" "A Exit"() -> (w1496:bool)
            }
          }
          frame #2 {
            n1348 = global write "Robot Global Data.vi" "A Drv"(FALSE ("Rumble")) -> ()
            n1349 = global write "Robot Global Data.vi" "A Exit"(FALSE ("Rumble")) -> ()
            n1350 = global write "Robot Global Data.vi" "VY Align"(FALSE ("VX Align")) -> ()
            n1351 = global write "Robot Global Data.vi" "Centering"(FALSE ("Centering")) -> ()
          }
        }
      }
    }
    n1352 = Wait (ms)(milliseconds to wait=u32 100) -> ()  [unwired: 1 out]
  }
